vi "Multi_Emitter_transmitter_ui.vi"() -> ()   [LabVIEW 2021]
uses:
  <vilib>/userdefined/High Color/nirio_resource_hc.ctl
  random_limits.ctl
  emitter params.ctl
  mode_type.ctl
  secnario config.ctl
  <instrlib>/niUsrpRio/Config/v1/Host/Public/niUsrpRio Session.ctl
  <instrlib>/_niInstr/Register Bus/v0/Host/Public/Register Bus Session.ctl
  <instrlib>/_niInstr/Register Bus/v0/Host/Private/Session Data.ctl
  <instrlib>/niUsrpRio/Config/v1/Host/Private/DB Queue Reference.ctl
  <instrlib>/niUsrpRio/Config/v1/Host/Private/Daughterboard Data.ctl
  <instrlib>/niUsrpRio/Config/v1/Host/Private/ATR state data.ctl
  <instrlib>/niUsrpRio/Config/v1/Host/Private/Antenna Configuration.ctl
  <instrlib>/niUsrpRio/Config/v1/Host/Private/CPLD Power Mode.ctl
  <instrlib>/niUsrpRio/Config/v1/Host/Public/EEPROM Header.ctl
  <instrlib>/niUsrpRio/Config/v1/Host/Public/EEPROM Device Data Header.ctl
  <instrlib>/niUsrpRio/Config/v1/Host/Public/EEPROM Characterization Header.ctl
  <instrlib>/niUsrpRio/Config/v1/Host/Public/Characterization Data.ctl
  <instrlib>/niUsrpRio/Config/v1/Host/Public/IQ Imbalance.ctl
  <instrlib>/niUsrpRio/Config/v1/Host/niUsrpRio Config v1 Host.lvlib
  <instrlib>/_niInstr/Register Bus/v0/Host/niInstr Register Bus v0 Host.lvlib
panel:
  out "String":string="Transmitting"
  in  "stop":bool=TRUE
  out "Pulse transmited":u32=20 format="%#.1p"
  out "FPGA clock":dbl=0.00084621 format="%#.1g"
  out "lost sampels - P2P":u32
  in  "Tab Control 2":enum32{"RF", "FPGA device", "VST", "TDMS files"}(tab)=enum."TDMS files"
  in  "RF gain":dbl=10.0 min=-130.0 max=30.0 format="%#.8p"
  in  "Center frequency (Hz)":dbl=1600000000.0 format="%#.8p"
  in  "P2P sample rate":dbl=200000000.0 format="%#.8p"
  in  "gen for DF":bool=TRUE
  in  "devicess":T1[](array[typedef])=["IF_transiver_0", "IF_transiver_1", "IF_transiver_2"]
  in  "vst_device":refnum<k15>[](array[refnum])
  in  "file paths":path[](array[path])=[path "C:/Users/PXIe8108_Demo/Documents/CHAIM DATA/chaim/5785_sync_for_elbit/data/pdw_test_file.tdms", path "C:/Users/PXIe8108_Demo/Documents/CHAIM DATA/chaim/5785_sync_for_elbit/data/pdw_test_file_1.tdms", path "C:/Users/PXIe8108_Demo/Documents/CHAIM DATA/chaim/5785_sync_for_elbit/data/pdw_test_file_2.tdms", path "C:/Users/PXIe8108_Demo/Documents/CHAIM DATA/chaim/5785_sync_for_elbit/data/pdw_test_file_3.tdms", path "C:/Users/PXIe8108_Demo/Documents/CHAIM DATA/chaim/5785_sync_for_elbit/data/pdw_test_file_4.tdms"]
  in  "Tab Control":T2(tab)=enum."Present scenario"
  in  "Tab Control 3":T3(tab)
  in  "rand limits":T4={"# Number of emitters"=84, "# Number of frequency per emitter"={"Numeric"=0, "Numeric"=22}, "Frequency range"={"Numeric"=158778625.95419848, "Numeric"=2894656488.5496182}, "Frequency dispersion for each emitter"={"Numeric"=0.0, "Numeric"=1181732.2396298076}, "PRI range (Hz)"={"Numeric"=33.59056776941936, "Numeric"=576.0533087800792}, "Duty cycle - pulse in PRI"={"Numeric"=0.026717557251908396, "Numeric"=0.11832061068702289}, "Amplitude (dB)"={"Numeric"=-34.62595419847328, "Numeric"=-51.11450381679389}, "Modulation depth"={"Numeric"=19162.08437325717, "Numeric"=1181732.2396298076}, "CW"=TRUE, "LFM"=TRUE, "DOA (DEG)"={"Numeric"=0.0, "Numeric"=1181732.2396298076}, "start time (Sec)"=0.0, "end time (Sec)"=50.0, "BPSK"=TRUE, "QPSK"=TRUE} {"DOA (DEG)" scale=0.0..360.0 scale format="%#_6f"; "Modulation depth" scale=1000.0..10000000.0 scale format="%#_6pHz"; "Amplitude (dB)" scale format="%#_6fdB"; "Duty cycle - pulse in PRI" scale=0.0..1.0 scale format="%#_6f"; "PRI range (Hz)" scale=1.0..3000.0 scale format="%#_6pHz"; "Frequency dispersion for each emitter" scale=1000000.0..100000000.0 scale format="%#_6pHz"; "Frequency range" scale=0.0..3200000000.0 scale format="%#_4pHz"; "# Number of frequency per emitter" scale=0.01..3000.0; "# Number of emitters" scale=0.0..200.0}
  in  "array":T5[](array[typedef]) {"t end" format="%#_13g"; "t start" format="%#_13g"; "DOA" format="%#_13g"; "mod depth" format="%#_13pHz"; "amp (dB)" format="%#_13gdB"; "d.c." format="%#_13g"; "hop rate (Hz)" format="%#_13pHz"; "f set" format="%#_6pHz"}
  in  "CSV pulse istraction file in":path=path "C:/Users/PXIe8108_Demo/Documents/CHAIM DATA/chaim/5785_sync_for_elbit/data/pdw_test_file_1.tdms"
  in  "Max number of pulses to present":dbl=500.0
  out "XY Graph":cluster{dbl[], dbl[]}[](graph)=[{[1580800140.0831814, 1580834407.004329], [6.623e-05, 0.00030966]}, {[2383313491.167746, 2383313491.167746], [9.1475e-05, 0.00041018]}, {[196157871.7414, 196805210.53311396], [0.000129485, 0.00029614500000000005]}, {[2893890730.2313623, 2893890730.2313623], [0.00020334, 0.000442945]}, {[2274621870.692988, 2274833527.2774396], [0.000263365, 0.00034213500000000003]}, {[826892720.0215597, 826892720.0215597, 826856448.7121654, 826856448.7121654, 826892720.0215597], [0.00034249, 0.000492215, 0.000492215, 0.00034249, 0.00034249]}, {[1739036854.6760328, 1739036854.6760328], [0.00034619, 0.000488535]}, {[1631334018.3591099, 1631334018.3591099, 1630358408.6030123, 1630358408.6030123, 1631334018.3591099], [0.000347855, 0.000533475, 0.000533475, 0.000347855, 0.000347855]}, {[2708416399.3761177, 2708416399.3761177, 2707616399.3761177, 2707616399.3761177, 2708416399.3761177], [0.00037931, 0.00062138, 0.00062138, 0.00037931, 0.00037931]}, {[2721351197.2689962, 2721351197.2689962, 2720538189.138915, 2720538189.138915, 2721351197.2689962], [0.000498795, 0.00067544, 0.00067544, 0.000498795, 0.000498795]}, {[680656193.5764762, 680656193.5764762], [0.000538285, 0.00082268]}, {[1109531948.6082644, 1109847037.660461], [0.000556095, 0.000896965]}, {[649464539.7076397, 649464539.7076397], [0.000556285, 0.000904715]}, {[2296419656.6224246, 2296419656.6224246], [0.000587275, 0.000693175]}, {[285702284.61423993, 285848939.51949644], [0.00059919, 0.00067695]}, {[1664070770.7339468, 1664070770.7339468, 1663177913.5910895, 1663177913.5910895, 1664070770.7339468], [0.000603985, 0.000816455, 0.000816455, 0.000603985, 0.000603985]}, {[1468598375.6912947, 1468823255.9824655], [0.000646, 0.000855]}, {[2866140899.355443, 2866140899.355443, 2866111509.201144, 2866111509.201144, 2866140899.355443], [0.00074212, 0.001017615, 0.001017615, 0.00074212, 0.00074212]}, {[1368139375.4725895, 1368139375.4725895, 1367154153.7977128, 1367154153.7977128, 1368139375.4725895], [0.000760645, 0.0009064850000000001, 0.0009064850000000001, 0.000760645, 0.000760645]}, {[2603761234.0340424, 2603761234.0340424, 2603302518.4377117, 2603302518.4377117, 2603761234.0340424], [0.00084391, 0.0009991, 0.0009991, 0.00084391, 0.00084391]}, {[472591034.81729984, 472591034.81729984, 472243208.73034334, 472243208.73034334, 472591034.81729984], [0.00086232, 0.00102511, 0.00102511, 0.00086232, 0.00086232]}, {[2879515070.2265687, 2879515070.2265687], [0.000892085, 0.0009666900000000001]}, {[1930031751.255956, 1930634378.2083786], [0.000947115, 0.001243875]}, {[2544253790.7099447, 2544253790.7099447], [0.000951505, 0.0010972]}, {[1824977446.8380158, 1824977446.8380158, 1823987347.828115, 1823987347.828115, 1824977446.8380158], [0.000955035, 0.00103088, 0.00103088, 0.000955035, 0.000955035]}, {[2202964376.3055444, 2202964376.3055444, 2202186166.1888127, 2202186166.1888127, 2202964376.3055444], [0.0009579, 0.001077815, 0.001077815, 0.0009579, 0.0009579]}, {[1514007725.1357243, 1514007725.1357243, 1513539341.060783, 1513539341.060783, 1514007725.1357243], [0.00098325, 0.001212565, 0.001212565, 0.00098325, 0.00098325]}, {[1450681049.292892, 1450681049.292892, 1450119251.5400832, 1450119251.5400832, 1450681049.292892], [0.00101241, 0.0012355, 0.0012355, 0.00101241, 0.00101241]}, {[2681398475.993289, 2681398475.993289, 2680255618.8504314, 2680255618.8504314, 2681398475.993289], [0.001092585, 0.00117186, 0.00117186, 0.001092585, 0.001092585]}, {[1407325102.8832715, 1407650065.0646722], [0.00117266, 0.001376915]}, {[646502856.5768648, 646502856.5768648], [0.00125212, 0.00135483]}, {[1489552387.630272, 1489552387.630272], [0.001275415, 0.001473835]}, {[1592242637.762581, 1592242637.762581], [0.00130457, 0.001472255]}, {[2395186268.257005, 2395186268.257005, 2394895570.582587, 2394895570.582587, 2395186268.257005], [0.00131468, 0.00202553, 0.00202553, 0.00131468, 0.00131468]}, {[894570399.7736647, 894570399.7736647, 893506569.9864306, 893506569.9864306, 894570399.7736647], [0.001317945, 0.001874215, 0.001874215, 0.001317945, 0.001317945]}, {[1705881079.1196365, 1705881079.1196365, 1705857272.4299567, 1705857272.4299567, 1705881079.1196365], [0.001409715, 0.00157576, 0.00157576, 0.001409715, 0.001409715]}, {[2251811039.783873, 2251811039.783873, 2251465616.6405225, 2251465616.6405225, 2251811039.783873], [0.001418575, 0.0014936700000000001, 0.0014936700000000001, 0.001418575, 0.001418575]}, {[2401581298.9745655, 2401646895.871443], [0.00142865, 0.001685845]}, {[549553368.0452126, 549553368.0452126], [0.00145178, 0.00166124]}, {[2845740333.033058, 2845740333.033058, 2845069192.093461, 2845069192.093461, 2845740333.033058], [0.0014714, 0.001763465, 0.001763465, 0.0014714, 0.0014714]}, {[997439632.3541692, 997439632.3541692, 997284833.5925595, 997284833.5925595, 997439632.3541692], [0.0015398, 0.001599625, 0.001599625, 0.0015398, 0.0015398]}, {[740736791.4399742, 740959489.4445376], [0.00172415, 0.00189051]}, {[1442023755.261369, 1442023755.261369, 1440954236.5447915, 1440954236.5447915, 1442023755.261369], [0.0017555, 0.0018244749999999999, 0.0018244749999999999, 0.0017555, 0.0017555]}, {[1449379123.164526, 1449379123.164526, 1449227031.9097729, 1449227031.9097729, 1449379123.164526], [0.00178903, 0.0019603900000000002, 0.0019603900000000002, 0.00178903, 0.00178903]}, {[2151473509.0573254, 2152401104.397768], [0.0017976, 0.0019175249999999998]}, {[771759513.8533624, 772735054.2043267], [0.00181764, 0.00195174]}, {[734571862.4124402, 734571862.4124402], [0.001888725, 0.00207308]}, {[196434462.20135283, 197081800.9930668], [0.001936905, 0.002103565]}, {[2800033039.6975074, 2800033039.6975074], [0.001991115, 0.002089685]}, {[1037674689.0691891, 1037674689.0691891, 1037232211.1930828, 1037232211.1930828, 1037674689.0691891], [0.0022019, 0.0023216350000000003, 0.0023216350000000003, 0.0022019, 0.0022019]}, {[1739062096.239286, 1739062096.239286], [0.002213105, 0.00235545]}, {[348761421.06253767, 348761421.06253767, 347856443.68697214, 347856443.68697214, 348761421.06253767], [0.00221368, 0.00258762, 0.00258762, 0.00221368, 0.00221368]}, {[1925417085.794845, 1925417085.794845], [0.00224428, 0.0025514]}, {[2774160892.4472075, 2774160892.4472075], [0.00226447, 0.0024049600000000003]}, {[2274272054.817277, 2274483711.4017286], [0.00226901, 0.0023477800000000003]}, {[592303104.7088935, 592303104.7088935, 591153679.4215372, 591153679.4215372, 592303104.7088935], [0.002297105, 0.002712025, 0.002712025, 0.002297105, 0.002297105]}, {[2296457382.3406115, 2296457382.3406115], [0.00232635, 0.00243225]}, {[1631268767.3701253, 1631268767.3701253, 1630293157.6140277, 1630293157.6140277, 1631268767.3701253], [0.00237092, 0.00255654, 0.00255654, 0.00237092, 0.00237092]}, {[1737912209.7280185, 1737912209.7280185, 1737388649.5185945, 1737388649.5185945, 1737912209.7280185], [0.00240274, 0.00291464, 0.00291464, 0.00240274, 0.00240274]}, {[1580608219.0446887, 1580642485.9658363], [0.002404205, 0.0026476349999999997]}, {[2721331571.011342, 2721331571.011342, 2720518562.881261, 2720518562.881261, 2721331571.011342], [0.0024361, 0.002612745, 0.002612745, 0.0024361, 0.0024361]}, {[1684929790.2362854, 1684929790.2362854, 1684531383.8617835, 1684531383.8617835, 1684929790.2362854], [0.002441555, 0.0026711900000000004, 0.0026711900000000004, 0.002441555, 0.002441555]}, {[1409155349.303642, 1409155349.303642, 1408497454.5667999, 1408497454.5667999, 1409155349.303642], [0.00252089, 0.002924655, 0.002924655, 0.00252089, 0.00252089]}, {[472660746.49775314, 472660746.49775314, 472312920.41079664, 472312920.41079664, 472660746.49775314], [0.00261325, 0.00277604, 0.00277604, 0.00261325, 0.00261325]}, {[2544181526.819716, 2544181526.819716], [0.00270404, 0.002849735]}, {[2893798188.6703253, 2893798188.6703253], [0.00271437, 0.0029539749999999997]}, {[1063127836.7713614, 1063127836.7713614, 1063048785.3879621, 1063048785.3879621, 1063127836.7713614], [0.002715655, 0.00316565, 0.00316565, 0.002715655, 0.002715655]}, {[2879351416.449822, 2879351416.449822], [0.002725625, 0.0028002300000000003]}, {[191171643.50208235, 191171643.50208235, 190384241.927279, 190384241.927279, 191171643.50208235], [0.00278627, 0.003685405, 0.003685405, 0.00278627, 0.00278627]}, {[1367987460.759361, 1367987460.759361, 1367002239.084484, 1367002239.084484, 1367987460.759361], [0.00280891, 0.00295475, 0.00295475, 0.00280891, 0.00280891]}, {[1824780231.2217734, 1824780231.2217734, 1823790132.2118726, 1823790132.2118726, 1824780231.2217734], [0.002821275, 0.00289712, 0.00289712, 0.002821275, 0.002821275]}, {[2880535219.9598703, 2880535219.9598703], [0.003022575, 0.003540315]}, {[285702284.61423993, 285848939.51949644], [0.00302315, 0.00310091]}, {[1513974483.6750598, 1513974483.6750598, 1513506099.6001184, 1513506099.6001184, 1513974483.6750598], [0.003061055, 0.00329037, 0.00329037, 0.003061055, 0.003061055]}, {[1468527568.6407409, 1468752448.9319117], [0.003138895, 0.003347895]}, {[1705219936.9474678, 1705219936.9474678, 1705196130.257788, 1705196130.257788, 1705219936.9474678], [0.003268275, 0.0034343200000000003, 0.0034343200000000003, 0.003268275, 0.003268275]}, {[1450726250.7121127, 1450726250.7121127, 1450164452.9593036, 1450164452.9593036, 1450726250.7121127], [0.003349665, 0.003572755, 0.003572755, 0.003349665, 0.003349665]}, {[1592373712.2870533, 1592373712.2870533], [0.003379285, 0.00354697]}, {[2202953811.6672707, 2202953811.6672707, 2202175601.550539, 2202175601.550539, 2202953811.6672707], [0.003414445, 0.00353436, 0.00353436, 0.003414445, 0.003414445]}, {[767132097.2802391, 767132097.2802391], [0.00341494, 0.00354653]}, {[1407300380.5714734, 1407625342.7528741], [0.003418365, 0.00362262]}, {[1663727218.3677917, 1663727218.3677917, 1662834361.2249343, 1662834361.2249343, 1663727218.3677917], [0.003432045, 0.003644515, 0.003644515, 0.003432045, 0.003432045]}, {[646535048.6960233, 646535048.6960233], [0.00347894, 0.0035816499999999996]}, {[2501631196.736514, 2501631196.736514, 2500683329.437936, 2500683329.437936, 2501631196.736514], [0.00352081, 0.004239565, 0.004239565, 0.00352081, 0.00352081]}, {[2603498435.1787024, 2603498435.1787024, 2603039719.5823717, 2603039719.5823717, 2603498435.1787024], [0.003578685, 0.0037338749999999998, 0.0037338749999999998, 0.003578685, 0.003578685]}, {[576427464.193527, 576427464.193527, 576181461.7335024, 576181461.7335024, 576427464.193527], [0.00358565, 0.004468335, 0.004468335, 0.00358565, 0.00358565]}, {[771327416.7103804, 772302957.0613447], [0.003643325, 0.003777425]}, {[2681146361.145378, 2681146361.145378, 2680003504.0025215, 2680003504.0025215, 2681146361.145378], [0.00369744, 0.0037767150000000004, 0.0037767150000000004, 0.00369744, 0.00369744]}, {[997064784.9392573, 997064784.9392573, 996909986.1776475, 996909986.1776475, 997064784.9392573], [0.00370627, 0.0037660949999999997, 0.0037660949999999997, 0.00370627, 0.00370627]}, {[1441877832.6486635, 1441877832.6486635, 1440808313.932086, 1440808313.932086, 1441877832.6486635], [0.003709485, 0.0037784600000000004, 0.0037784600000000004, 0.003709485, 0.003709485]}, {[1184679216.2804806, 1184679216.2804806, 1184560662.6349561, 1184560662.6349561, 1184679216.2804806], [0.003714075, 0.003895875, 0.003895875, 0.003714075, 0.003714075]}, {[549553368.0452126, 549553368.0452126], [0.00371751, 0.00392697]}, {[2865958264.9593143, 2865958264.9593143, 2865928874.8050165, 2865928874.8050165, 2865958264.9593143], [0.00372947, 0.004004965, 0.004004965, 0.00372947, 0.00372947]}, {[196469763.70549965, 197117102.4972136], [0.00374432, 0.0039109800000000005]}, {[1449313379.2357452, 1449313379.2357452, 1449161287.9809923, 1449161287.9809923, 1449313379.2357452], [0.003774055, 0.003945415, 0.003945415, 0.003774055, 0.003774055]}, {[2252044360.969656, 2252044360.969656, 2251698937.8263054, 2251698937.8263054, 2252044360.969656], [0.003835815, 0.00391091, 0.00391091, 0.003835815, 0.003835815]}, {[2754483678.838529, 2754483678.838529, 2753805712.736834, 2753805712.736834, 2754483678.838529], [0.00384677, 0.004098795, 0.004098795, 0.00384677, 0.00384677]}, {[952948653.5105207, 952948653.5105207], [0.003865105, 0.004472745]}, {[2151381942.365458, 2152309537.7059007], [0.0039314, 0.004051325]}, {[2383187284.4591317, 2383187284.4591317], [0.00394438, 0.004263085]}, {[2296696866.079333, 2296696866.079333], [0.00406542, 0.00417132]}, {[1739061006.477425, 1739061006.477425], [0.00408002, 0.0042223650000000005]}, {[826977891.3539693, 826977891.3539693, 826941620.044575, 826941620.044575, 826977891.3539693], [0.004121665, 0.00427139, 0.00427139, 0.004121665, 0.004121665]}, {[734773527.9249377, 734773527.9249377], [0.00414752, 0.004331875]}, {[740723871.5179688, 740946569.5225322], [0.004163125, 0.004329485]}, {[2708532448.1508884, 2708532448.1508884, 2707732448.1508884, 2707732448.1508884, 2708532448.1508884], [0.00421376, 0.00445583, 0.00445583, 0.00421376, 0.00421376]}, {[2800458079.9117093, 2800458079.9117093], [0.00423334, 0.0043319100000000004]}, {[2274666375.3677125, 2274878031.952164], [0.00427466, 0.004353429999999999]}, {[1930166193.4840126, 1930768820.4364355], [0.00435341, 0.00465017]}, {[472726219.80381584, 472726219.80381584, 472378393.71685934, 472378393.71685934, 472726219.80381584], [0.004364175, 0.004526965, 0.004526965, 0.004364175, 0.004364175]}, {[513973938.6140039, 513973938.6140039, 513160930.4839227, 513160930.4839227, 513973938.6140039], [0.00437234, 0.00503197, 0.00503197, 0.00437234, 0.00437234]}, {[2720887898.354795, 2720887898.354795, 2720074890.224714, 2720074890.224714, 2720887898.354795], [0.004373405, 0.00455005, 0.00455005, 0.004373405, 0.004373405]}, {[1631196040.4311666, 1631196040.4311666, 1630220430.675069, 1630220430.675069, 1631196040.4311666], [0.004393985, 0.0045796050000000005, 0.0045796050000000005, 0.004393985, 0.004393985]}, {[2544196925.447932, 2544196925.447932], [0.004456575, 0.00460227]}, {[2879644419.775343, 2879644419.775343], [0.004559165, 0.00463377]}, {[648876109.0898465, 648876109.0898465, 648365905.0082139, 648365905.0082139, 648876109.0898465], [0.00460361, 0.0053656400000000005, 0.0053656400000000005, 0.00460361, 0.00460361]}, {[1109802779.3598022, 1110117868.4119987], [0.0046591, 0.00499997]}, {[1824895450.5609894, 1824895450.5609894, 1823905351.5510883, 1823905351.5510883, 1824895450.5609894], [0.00468751, 0.0047633549999999995, 0.0047633549999999995, 0.00468751, 0.00468751]}, {[1580945890.5906582, 1580980157.5118058], [0.004742185, 0.0049856150000000005]}, {[1437976628.2282147, 1437976628.2282147, 1437095570.9594924, 1437095570.9594924, 1437976628.2282147], [0.00476518, 0.005106085, 0.005106085, 0.00476518, 0.00476518]}, {[1367912019.2469618, 1367912019.2469618, 1366926797.572085, 1366926797.572085, 1367912019.2469618], [0.00485718, 0.00500302, 0.00500302, 0.00485718, 0.00485718]}, {[2642546476.6451225, 2642546476.6451225], [0.005085275, 0.005440550000000001]}, {[2401764599.7099066, 2401830196.606784], [0.00512136, 0.005378555]}, {[1706050956.0580258, 1706050956.0580258, 1706027149.368346, 1706027149.368346, 1706050956.0580258], [0.00512683, 0.005292875, 0.005292875, 0.00512683, 0.00512683]}, {[1684720808.2794032, 1684720808.2794032, 1684322401.9049013, 1684322401.9049013, 1684720808.2794032], [0.00513206, 0.005361695, 0.005361695, 0.00513206, 0.00513206]}, {[1513882285.9166286, 1513882285.9166286, 1513413901.8416872, 1513413901.8416872, 1513882285.9166286], [0.00513886, 0.005368175, 0.005368175, 0.00513886, 0.00513886]}, {[2549489795.642293, 2549489795.642293, 2549255329.0537815, 2549255329.0537815, 2549489795.642293], [0.00521551, 0.005773825, 0.005773825, 0.00521551, 0.00521551]}, {[2893775785.8287454, 2893775785.8287454], [0.005225405, 0.00546501]}, {[1925417085.794845, 1925417085.794845], [0.00527129, 0.00557841]}, {[2773799782.619938, 2773799782.619938], [0.005372855, 0.005513345]}, {[285702284.61423993, 285848939.51949644], [0.005447115, 0.005524874999999999]}, {[1591792582.9263594, 1591792582.9263594], [0.005454, 0.0056216849999999995]}, {[771543002.2032365, 772518542.5542008], [0.005469015, 0.005603115]}, {[1662007237.9519308, 1662007237.9519308, 1661585297.023661, 1661585297.023661, 1662007237.9519308], [0.005534915, 0.005872784999999999, 0.005872784999999999, 0.005534915, 0.005534915]}, {[196056287.52977967, 196703626.32149363], [0.005551735, 0.005718395]}, {[1037437198.7534403, 1037437198.7534403, 1036994720.877334, 1036994720.877334, 1037437198.7534403], [0.005624565, 0.0057443, 0.0057443, 0.005624565, 0.005624565]}, {[1469056690.8281426, 1469281571.1193135], [0.00563179, 0.00584079]}, {[1441880281.2689369, 1441880281.2689369, 1440810762.5523593, 1440810762.5523593, 1441880281.2689369], [0.00566347, 0.005732445, 0.005732445, 0.00566347, 0.00566347]}, {[1407344576.5288398, 1407669538.7102404], [0.00566407, 0.005868325000000001]}, {[1450710289.7500644, 1450710289.7500644, 1450148491.9972553, 1450148491.9972553, 1450710289.7500644], [0.00568692, 0.00591001, 0.00591001, 0.00568692, 0.00568692]}, {[646220455.0854722, 646220455.0854722], [0.00570576, 0.00580847]}, {[1449379123.164526, 1449379123.164526, 1449227031.9097729, 1449227031.9097729, 1449379123.164526], [0.005759075, 0.0059304349999999995, 0.0059304349999999995, 0.005759075, 0.005759075]}, {[2296096376.8515058, 2296096376.8515058], [0.005804495, 0.005910395]}, {[2203062554.686778, 2203062554.686778, 2202284344.5700464, 2202284344.5700464, 2203062554.686778], [0.00587099, 0.005990905, 0.005990905, 0.00587099, 0.00587099]}, {[997192164.9389083, 997192164.9389083, 997037366.1772985, 997037366.1772985, 997192164.9389083], [0.005872745, 0.005932570000000001, 0.005932570000000001, 0.005872745, 0.005872745]}, {[1489463100.0648816, 1489463100.0648816], [0.00588631, 0.00608473]}, {[1738991102.0076396, 1738991102.0076396], [0.005946935, 0.006089280000000001]}, {[1409155349.303642, 1409155349.303642, 1408497454.5667999, 1408497454.5667999, 1409155349.303642], [0.005972975, 0.0063767400000000005, 0.0063767400000000005, 0.005972975, 0.005972975]}, {[549553368.0452126, 549553368.0452126], [0.00598324, 0.0061927]}, {[2151368361.287098, 2152295956.6275406], [0.006065195, 0.00618512]}, {[472451052.26250076, 472451052.26250076, 472103226.17554426, 472103226.17554426, 472451052.26250076], [0.006115105, 0.006277895, 0.006277895, 0.006115105, 0.006115105]}, {[894611310.8512297, 894611310.8512297, 893547481.0639956, 893547481.0639956, 894611310.8512297], [0.00611715, 0.00667342, 0.00667342, 0.00611715, 0.00611715]}, {[2544312914.5976286, 2544312914.5976286], [0.00620911, 0.006354805000000001]}, {[2251793159.6009665, 2251793159.6009665, 2251447736.457616, 2251447736.457616, 2251793159.6009665], [0.00625305, 0.006328144999999999, 0.006328144999999999, 0.00625305, 0.00625305]}, {[1663706181.7369223, 1663706181.7369223, 1662813324.5940652, 1662813324.5940652, 1663706181.7369223], [0.00626011, 0.00647258, 0.00647258, 0.00626011, 0.00626011]}, {[2274457073.9342976, 2274668730.518749], [0.006280305, 0.006359075]}, {[2681119550.8547864, 2681119550.8547864, 2679976693.7119293, 2679976693.7119293, 2681119550.8547864], [0.006302295, 0.0063815700000000005, 0.0063815700000000005, 0.006302295, 0.006302295]}, {[2721608626.7745028, 2721608626.7745028, 2720795618.6444216, 2720795618.6444216, 2721608626.7745028], [0.006310705, 0.006487349999999999, 0.006487349999999999, 0.006310705, 0.006310705]}, {[2603629941.7925797, 2603629941.7925797, 2603171226.196249, 2603171226.196249, 2603629941.7925797], [0.006313465, 0.006468655, 0.006468655, 0.006313465, 0.006313465]}, {[2232122993.202605, 2232122993.202605, 2231064792.144404, 2231064792.144404, 2232122993.202605], [0.006389155, 0.007933144999999999, 0.007933144999999999, 0.006389155, 0.006389155]}, {[2879383848.0123553, 2879383848.0123553], [0.0063927, 0.0064673050000000004]}, {[680656193.5764762, 680656193.5764762], [0.00639547, 0.006679865]}, {[734464036.7508987, 734464036.7508987], [0.00640632, 0.006590675]}, {[1631325077.6087675, 1631325077.6087675, 1630349467.85267, 1630349467.85267, 1631325077.6087675], [0.00641705, 0.00660267, 0.00660267, 0.00641705, 0.00641705]}, {[2800080381.365308, 2800080381.365308], [0.00647557, 0.00657414]}, {[1824943974.0034225, 1824943974.0034225, 1823953874.9935215, 1823953874.9935215, 1824943974.0034225], [0.006553745, 0.0066295899999999994, 0.0066295899999999994, 0.006553745, 0.006553745]}, {[740729002.861417, 740951700.8659805], [0.006602095, 0.006768455]}, {[592101558.0578947, 592101558.0578947, 590952132.7705383, 590952132.7705383, 592101558.0578947], [0.00665653, 0.00707145, 0.00707145, 0.00665653, 0.00665653]}, {[2866116016.872055, 2866116016.872055, 2866086626.717757, 2866086626.717757, 2866116016.872055], [0.00671682, 0.006992315, 0.006992315, 0.00671682, 0.00671682]}, {[358280471.4209943, 358280471.4209943, 357692236.12687683, 357692236.12687683, 358280471.4209943], [0.00684166, 0.00769989, 0.00769989, 0.00684166, 0.00684166]}, {[1368746211.5180047, 1368746211.5180047, 1367760989.8431277, 1367760989.8431277, 1368746211.5180047], [0.006905445, 0.007051285, 0.007051285, 0.006905445, 0.006905445]}, {[767335940.9524096, 767335940.9524096], [0.006929165, 0.007060755]}, {[1705193072.3917153, 1705193072.3917153, 1705169265.7020354, 1705169265.7020354, 1705193072.3917153], [0.006985385, 0.00715143, 0.00715143, 0.006985385, 0.006985385]}, {[1580759500.4395807, 1580793767.3607285], [0.00708016, 0.0073235900000000005]}, {[1513727389.6331923, 1513727389.6331923, 1513259005.558251, 1513259005.558251, 1513727389.6331923], [0.007216665, 0.00744598, 0.00744598, 0.007216665, 0.007216665]}, {[771474197.2723118, 772449737.6232761], [0.0072947, 0.0074288]}, {[196593060.32748413, 197240399.11919808], [0.007359155, 0.007525815]}, {[1063299761.3303311, 1063299761.3303311, 1063220709.9469318, 1063220709.9469318, 1063299761.3303311], [0.00739398, 0.007843975, 0.007843975, 0.00739398, 0.00739398]}, {[2395319994.632628, 2395319994.632628, 2395029296.958209, 2395029296.958209, 2395319994.632628], [0.007472035, 0.008182885, 0.008182885, 0.007472035, 0.007472035]}, {[1591840538.1910703, 1591840538.1910703], [0.007528715, 0.0076964]}, {[2296089760.628729, 2296089760.628729], [0.00754357, 0.00764947]}, {[2845678014.9449577, 2845678014.9449577, 2845006874.0053606, 2845006874.0053606, 2845678014.9449577], [0.0075644, 0.007856465, 0.007856465, 0.0075644, 0.0075644]}, {[1442860787.5168386, 1442860787.5168386, 1441791268.800261, 1441791268.800261, 1442860787.5168386], [0.007617455, 0.00768643, 0.00768643, 0.007617455, 0.007617455]}, {[2893859155.9198585, 2893859155.9198585], [0.007736435, 0.00797604]}, {[1449313379.2357452, 1449313379.2357452, 1449161287.9809923, 1449161287.9809923, 1449313379.2357452], [0.007744095, 0.007915455, 0.007915455, 0.007744095, 0.007744095]}, {[1929892018.70746, 1930494645.6598828], [0.007759705, 0.008056465]}, {[2383333327.4941196, 2383333327.4941196], [0.007797285, 0.00811599]}, {[1738987303.8463974, 1738987303.8463974], [0.00781385, 0.007956195000000001]}, {[1684959175.0429544, 1684959175.0429544, 1684560768.6684525, 1684560768.6684525, 1684959175.0429544], [0.007822565, 0.0080522, 0.0080522, 0.007822565, 0.007822565]}, {[472589383.96592045, 472589383.96592045, 472241557.87896395, 472241557.87896395, 472589383.96592045], [0.00786603, 0.008028819999999999, 0.008028819999999999, 0.00786603, 0.00786603]}, {[285702284.61423993, 285848939.51949644], [0.007871075, 0.007948835]}, {[826842646.1959547, 826842646.1959547, 826806374.8865603, 826806374.8865603, 826842646.1959547], [0.00790084, 0.008050564999999999, 0.008050564999999999, 0.00790084, 0.00790084]}, {[1407289616.8067927, 1407614578.9881935], [0.00790977, 0.008114025]}, {[646574240.5246942, 646574240.5246942], [0.007932575, 0.008035285000000001]}, {[2544396206.6976385, 2544396206.6976385], [0.00796164, 0.008107335]}, {[1450589789.1001937, 1450589789.1001937, 1450027991.3473847, 1450027991.3473847, 1450589789.1001937], [0.008024175, 0.008247265, 0.008247265, 0.008024175, 0.008024175]}, {[997068963.0170933, 997068963.0170933, 996914164.2554835, 996914164.2554835, 997068963.0170933], [0.00803922, 0.008099045, 0.008099045, 0.00803922, 0.00803922]}, {[1184681571.1905012, 1184681571.1905012, 1184563017.5449767, 1184563017.5449767, 1184681571.1905012], [0.00804374, 0.00822554, 0.00822554, 0.00804374, 0.00804374]}, {[2708441543.4714837, 2708441543.4714837, 2707641543.4714837, 2707641543.4714837, 2708441543.4714837], [0.00804821, 0.00829028, 0.00829028, 0.00804821, 0.00804821]}, {[1468945567.8784726, 1469170448.1696434], [0.00812469, 0.008333690000000001]}, {[2317953472.4606924, 2317953472.4606924], [0.008127065, 0.010070595]}, {[2151428965.0152593, 2152356560.355702], [0.008198995, 0.00831892]}, {[348658294.97384024, 348658294.97384024, 347753317.5982747, 347753317.5982747, 348658294.97384024], [0.00822505, 0.008598989999999999, 0.008598989999999999, 0.00822505, 0.00822505]}, {[2879290525.343538, 2879290525.343538], [0.00822624, 0.008300845]}, {[2721648319.4452286, 2721648319.4452286, 2720835311.3151474, 2720835311.3151474, 2721648319.4452286], [0.00824801, 0.008424655, 0.008424655, 0.00824801, 0.00824801]}, {[549553368.0452126, 549553368.0452126], [0.008248965, 0.008458425]}, {[2274181451.318759, 2274393107.9032106], [0.008285955, 0.008364725]}, {[1925417085.794845, 1925417085.794845], [0.008298295, 0.008605415]}, {[2203696245.445428, 2203696245.445428, 2202918035.3286963, 2202918035.3286963, 2203696245.445428], [0.00832753, 0.008447445, 0.008447445, 0.00832753, 0.00832753]}, {[2234822554.778743, 2234822554.778743, 2233967853.9240417, 2233967853.9240417, 2234822554.778743], [0.00838687, 0.009563084999999999, 0.009563084999999999, 0.00838687, 0.00838687]}, {[1824774748.6669872, 1824774748.6669872, 1823784649.6570861, 1823784649.6570861, 1824774748.6669872], [0.00841998, 0.008495825, 0.008495825, 0.00841998, 0.00841998]}, {[1631352666.923056, 1631352666.923056, 1630377057.1669583, 1630377057.1669583, 1631352666.923056], [0.008440115, 0.008625734999999999, 0.008625734999999999, 0.008440115, 0.008440115]}, {[2774131413.6681013, 2774131413.6681013], [0.00848124, 0.00862173]}, {[2880970854.8082085, 2880970854.8082085], [0.008508115, 0.009025855]}, {[734700021.0995475, 734700021.0995475], [0.008665115, 0.00884947]}, {[2252003552.7850003, 2252003552.7850003, 2251658129.6416497, 2251658129.6416497, 2252003552.7850003], [0.00867029, 0.008745385000000001, 0.008745385000000001, 0.00867029, 0.00867029]}, {[2800025632.1998563, 2800025632.1998563], [0.008717795, 0.008816365]}, {[1109761244.8834865, 1110076333.935683], [0.00876211, 0.00910298]}, {[2402109882.815182, 2402175479.712059], [0.008814065, 0.00907126]}, {[1705327327.5286741, 1705327327.5286741, 1705303520.8389943, 1705303520.8389943, 1705327327.5286741], [0.00884394, 0.009009985, 0.009009985, 0.00884394, 0.00884394]}, {[2681025969.7430334, 2681025969.7430334, 2679883112.6001763, 2679883112.6001763, 2681025969.7430334], [0.00890715, 0.008986425000000001, 0.008986425000000001, 0.00890715, 0.00890715]}, {[1368691160.8756483, 1368691160.8756483, 1367705939.2007713, 1367705939.2007713, 1368691160.8756483], [0.008953715, 0.009099554999999999, 0.009099554999999999, 0.008953715, 0.008953715]}, {[2755073705.6039343, 2755073705.6039343, 2754395739.502239, 2754395739.502239, 2755073705.6039343], [0.009011195, 0.009263219999999999, 0.009263219999999999, 0.009011195, 0.009011195]}, {[740893521.581745, 741116219.5863085], [0.00904107, 0.00920743]}, {[1037849812.9642878, 1037849812.9642878, 1037407335.0881815, 1037407335.0881815, 1037849812.9642878], [0.009047235, 0.00916697, 0.00916697, 0.009047235, 0.009047235]}, {[2603575983.0110044, 2603575983.0110044, 2603117267.414674, 2603117267.414674, 2603575983.0110044], [0.00904824, 0.00920343, 0.00920343, 0.00904824, 0.00904824]}, {[1663658939.9626198, 1663658939.9626198, 1662766082.8197625, 1662766082.8197625, 1663658939.9626198], [0.00908817, 0.009300639999999999, 0.009300639999999999, 0.00908817, 0.00908817]}, {[771369562.2871455, 772345102.6381098], [0.009120385, 0.009254485]}, {[196558768.56656957, 197206107.35828352], [0.00916657, 0.009333230000000001]}, {[2296716536.6770926, 2296716536.6770926], [0.00928264, 0.00938854]}, {[1513642762.6943433, 1513642762.6943433, 1513174378.619402, 1513174378.619402, 1513642762.6943433], [0.009294465, 0.00952378, 0.00952378, 0.009294465, 0.009294465]}, {[1580885021.106201, 1580919288.0273485], [0.009418135, 0.009661564999999999]}, {[1409155349.303642, 1409155349.303642, 1408497454.5667999, 1408497454.5667999, 1409155349.303642], [0.00942506, 0.009828825000000001, 0.009828825000000001, 0.00942506, 0.00942506]}, {[1442388293.9242394, 1442388293.9242394, 1441318775.2076619, 1441318775.2076619, 1442388293.9242394], [0.00957144, 0.009640415000000001, 0.009640415000000001, 0.00957144, 0.00957144]}, {[1592106085.5720952, 1592106085.5720952], [0.00960343, 0.009771115]}, {[472872663.51137424, 472872663.51137424, 472524837.42441773, 472524837.42441773, 472872663.51137424], [0.00961696, 0.00977975, 0.00977975, 0.00961696, 0.00961696]}, {[1739056589.8570004, 1739056589.8570004], [0.009680765, 0.00982311]}, {[2865918129.068333, 2865918129.068333, 2865888738.914035, 2865888738.914035, 2865918129.068333], [0.00970417, 0.009979665, 0.009979665, 0.00970417, 0.00970417]}, {[2544131870.074193, 2544131870.074193], [0.009714175, 0.00985987]}, {[1737963778.3685791, 1737963778.3685791, 1737440218.1591551, 1737440218.1591551, 1737963778.3685791], [0.009719545, 0.010231444999999999, 0.010231444999999999, 0.009719545, 0.009719545]}, {[1449379123.164526, 1449379123.164526, 1449227031.9097729, 1449227031.9097729, 1449379123.164526], [0.009729115, 0.009900475, 0.009900475, 0.009729115, 0.009729115]}, {[953499027.9946896, 953499027.9946896], [0.009734975, 0.010342615]}, {[2879485571.71311, 2879485571.71311], [0.01005978, 0.010134385000000001]}, {[1407325102.8832715, 1407650065.0646722], [0.010155475, 0.010359730000000001]}, {[513660630.55560327, 513660630.55560327, 512847622.4255221, 512847622.4255221, 513660630.55560327], [0.01015609, 0.01081572, 0.01081572, 0.01015609, 0.01015609]}, {[646084411.6524413, 646084411.6524413], [0.010159395, 0.010262105]}, {[2721571531.409893, 2721571531.409893, 2720758523.279812, 2720758523.279812, 2721571531.409893], [0.010185315, 0.01036196, 0.01036196, 0.010185315, 0.010185315]}, {[997428634.6466807, 997428634.6466807, 997273835.8850709, 997273835.8850709, 997428634.6466807], [0.010205695, 0.01026552, 0.01026552, 0.010205695, 0.010205695]}, {[2893835322.437974, 2893835322.437974], [0.010247465, 0.010487070000000001]}, {[1824794220.2309835, 1824794220.2309835, 1823804121.2210824, 1823804121.2210824, 1824794220.2309835], [0.010286215, 0.01036206, 0.01036206, 0.010286215, 0.010286215]}, {[2273952247.704483, 2274163904.2889347], [0.0102916, 0.01037037]}, {[285702284.61423993, 285848939.51949644], [0.01029504, 0.0103728]}, {[2151478147.548687, 2152405742.8891296], [0.010332795, 0.01045272]}, {[1450601418.442362, 1450601418.442362, 1450039620.689553, 1450039620.689553, 1450601418.442362], [0.010361425, 0.010584515000000001, 0.010584515000000001, 0.010361425, 0.010361425]}, {[767010222.9587655, 767010222.9587655], [0.010443385, 0.010574975]}, {[1631375527.8903732, 1631375527.8903732, 1630399918.1342757, 1630399918.1342757, 1631375527.8903732], [0.010463175, 0.010648794999999999, 0.010648794999999999, 0.010463175, 0.010463175]}, {[1489671501.0283628, 1489671501.0283628], [0.01049721, 0.01069563]}, {[1685032737.4106975, 1685032737.4106975, 1684634331.0361953, 1684634331.0361953, 1685032737.4106975], [0.010513065, 0.0107427, 0.0107427, 0.010513065, 0.010513065]}, {[549553368.0452126, 549553368.0452126], [0.010514695, 0.010724154999999999]}, {[1468768186.1909142, 1468993066.482085], [0.010617585, 0.010826585000000001]}, {[649464539.7076397, 649464539.7076397], [0.010647545, 0.010995975]}, {[1705828281.0006616, 1705828281.0006616, 1705804474.3109818, 1705804474.3109818, 1705828281.0006616], [0.010702495, 0.01086854, 0.01086854, 0.010702495, 0.010702495]}, {[2203292231.878026, 2203292231.878026, 2202514021.761295, 2202514021.761295, 2203292231.878026], [0.010784075, 0.01090399, 0.01090399, 0.010784075, 0.010784075]}, {[894381668.9630754, 894381668.9630754, 893317839.1758413, 893317839.1758413, 894381668.9630754], [0.01091636, 0.01147263, 0.01147263, 0.01091636, 0.01091636]}, {[734686923.4632208, 734686923.4632208], [0.01092391, 0.011108265]}, {[771534875.8640743, 772510416.2150387], [0.010946075, 0.011080175]}, {[2800471429.041852, 2800471429.041852], [0.010960025, 0.011058595]}, {[196626663.36879516, 197274002.1605091], [0.010973985, 0.011140645000000001]}, {[1367892214.719479, 1367892214.719479, 1366906993.0446022, 1366906993.0446022, 1367892214.719479], [0.01100198, 0.01114782, 0.01114782, 0.01100198, 0.01100198]}, {[591753124.3896897, 591753124.3896897, 590603699.1023333, 590603699.1023333, 591753124.3896897], [0.011015955, 0.011430874999999998, 0.011430874999999998, 0.011015955, 0.011015955]}, {[2296311292.262669, 2296311292.262669], [0.011021715, 0.011127615]}, {[2252072419.0839663, 2252072419.0839663, 2251726995.9406157, 2251726995.9406157, 2252072419.0839663], [0.011087525, 0.011162620000000002, 0.011162620000000002, 0.011087525, 0.011087525]}, {[1930031751.255956, 1930634378.2083786], [0.011166, 0.01146276]}, {[1925417085.794845, 1925417085.794845], [0.0113253, 0.01163242]}, {[472591034.81729984, 472591034.81729984, 472243208.73034334, 472243208.73034334, 472591034.81729984], [0.011367885, 0.011530674999999999, 0.011530674999999999, 0.011367885, 0.011367885]}, {[1513665052.2554708, 1513665052.2554708, 1513196668.180529, 1513196668.180529, 1513665052.2554708], [0.01137227, 0.011601585000000001, 0.011601585000000001, 0.01137227, 0.01137227]}, {[2544191636.0495725, 2544191636.0495725], [0.01146671, 0.011612405]}, {[740788064.5607747, 741010762.5653381], [0.011480045, 0.011646405]}, {[2681398475.993289, 2681398475.993289, 2680255618.8504314, 2680255618.8504314, 2681398475.993289], [0.011512005, 0.01159128, 0.01159128, 0.011512005, 0.011512005]}, {[1441785058.2562668, 1441785058.2562668, 1440715539.5396893, 1440715539.5396893, 1441785058.2562668], [0.011525425, 0.011594400000000001, 0.011594400000000001, 0.011525425, 0.011525425]}, {[1739041782.8394334, 1739041782.8394334], [0.01154768, 0.011690025]}, {[2773676206.927871, 2773676206.927871], [0.011589625, 0.011730115]}, {[1662122651.5154796, 1662122651.5154796, 1661700710.5872097, 1661700710.5872097, 1662122651.5154796], [0.011627, 0.01196487, 0.01196487, 0.011627, 0.011627]}, {[2383159668.1059523, 2383159668.1059523], [0.01165019, 0.011968895]}, {[1592012680.4076858, 1592012680.4076858], [0.011678145, 0.01184583]}, {[826890425.1105181, 826890425.1105181, 826854153.8011237, 826854153.8011237, 826890425.1105181], [0.01168002, 0.011829745, 0.011829745, 0.01168002, 0.01168002]}, {[1449313379.2357452, 1449313379.2357452, 1449161287.9809923, 1449161287.9809923, 1449313379.2357452], [0.01171414, 0.0118855, 0.0118855, 0.01171414, 0.01171414]}, {[1581070751.4417686, 1581105018.3629162], [0.011756115, 0.011999544999999999]}, {[2603675335.7246003, 2603675335.7246003, 2603216620.12827, 2603216620.12827, 2603675335.7246003], [0.01178302, 0.01193821, 0.01193821, 0.01178302, 0.01178302]}, {[2708163722.6427097, 2708163722.6427097, 2707363722.6427097, 2707363722.6427097, 2708163722.6427097], [0.011882665, 0.012124735000000001, 0.012124735000000001, 0.011882665, 0.011882665]}, {[2879846973.8631067, 2879846973.8631067], [0.01189332, 0.011967925]}, {[1663627126.801152, 1663627126.801152, 1662734269.658295, 1662734269.658295, 1663627126.801152], [0.01191623, 0.0121287, 0.0121287, 0.01191623, 0.01191623]}, {[1063253930.5611609, 1063253930.5611609, 1063174879.1777617, 1063174879.1777617, 1063253930.5611609], [0.012072305, 0.0125223, 0.0125223, 0.012072305, 0.012072305]}, {[2721351197.2689962, 2721351197.2689962, 2720538189.138915, 2720538189.138915, 2721351197.2689962], [0.01212262, 0.012299265, 0.012299265, 0.01212262, 0.01212262]}, {[1824744659.720948, 1824744659.720948, 1823754560.7110472, 1823754560.7110472, 1824744659.720948], [0.01215245, 0.012228295, 0.012228295, 0.01215245, 0.01215245]}, {[680656193.5764762, 680656193.5764762], [0.01225265, 0.012537045]}, {[2274555327.372104, 2274766983.956556], [0.01229725, 0.01237602]}, {[996991553.1942685, 996991553.1942685, 996836754.4326587, 996836754.4326587, 996991553.1942685], [0.012372165, 0.012431989999999999, 0.012431989999999999, 0.012372165, 0.012372165]}, {[1184652956.373427, 1184652956.373427, 1184534402.7279022, 1184534402.7279022, 1184652956.373427], [0.012373405, 0.012555205, 0.012555205, 0.012373405, 0.012373405]}, {[646502856.5768648, 646502856.5768648], [0.012386215, 0.012488925000000001]}, {[1407300380.5714734, 1407625342.7528741], [0.01240118, 0.012605435]}, {[2643010540.7462864, 2643010540.7462864], [0.012452405, 0.01280768]}, {[2151502369.854427, 2152429965.1948695], [0.01246659, 0.012586515]}, {[1037638449.2997943, 1037638449.2997943, 1037195971.423688, 1037195971.423688, 1037638449.2997943], [0.0124699, 0.012589635, 0.012589635, 0.0124699, 0.0124699]}, {[1631390437.082894, 1631390437.082894, 1630414827.3267965, 1630414827.3267965, 1631390437.082894], [0.01248624, 0.012671859999999998, 0.012671859999999998, 0.01248624, 0.01248624]}, {[2401581298.9745655, 2401646895.871443], [0.012506775, 0.01276397]}, {[1705079320.2711687, 1705079320.2711687, 1705055513.581489, 1705055513.581489, 1705079320.2711687], [0.01256105, 0.012727095, 0.012727095, 0.01256105, 0.01256105]}, {[2865887879.658575, 2865887879.658575, 2865858489.5042768, 2865858489.5042768, 2865887879.658575], [0.01269152, 0.012967015, 0.012967015, 0.01269152, 0.01269152]}, {[1450690643.6663926, 1450690643.6663926, 1450128845.9135835, 1450128845.9135835, 1450690643.6663926], [0.01269868, 0.01292177, 0.01292177, 0.01269868, 0.01269868]}, {[285702284.61423993, 285848939.51949644], [0.012719, 0.012796759999999999]}, {[2893895761.2772584, 2893895761.2772584], [0.012758495, 0.0129981]}, {[2296605379.3567424, 2296605379.3567424], [0.012760785, 0.012866685000000001]}, {[771488196.8876398, 772463737.2386041], [0.01277176, 0.01290586]}, {[549553368.0452126, 549553368.0452126], [0.012780425, 0.012989885]}, {[195898497.85518265, 196545836.6468966], [0.012781405, 0.012948065]}, {[1437851190.719583, 1437851190.719583, 1436970133.4508605, 1436970133.4508605, 1437851190.719583], [0.01280003, 0.013140935000000001, 0.013140935000000001, 0.01280003, 0.01280003]}, {[1109829949.8347387, 1110145038.8869352], [0.01286512, 0.01320599]}, {[1409155349.303642, 1409155349.303642, 1408497454.5667999, 1408497454.5667999, 1409155349.303642], [0.01287714, 0.013280905, 0.013280905, 0.01287714, 0.01287714]}, {[1368466421.5023482, 1368466421.5023482, 1367481199.8274713, 1367481199.8274713, 1368466421.5023482], [0.01305025, 0.013196089999999999, 0.013196089999999999, 0.01305025, 0.01305025]}, {[1468372436.7318177, 1468597317.0229886], [0.01311048, 0.013319480000000002]}, {[472660746.49775314, 472660746.49775314, 472312920.41079664, 472312920.41079664, 472660746.49775314], [0.013118815, 0.013281605, 0.013281605, 0.013118815, 0.013118815]}, {[734531669.9672707, 734531669.9672707], [0.013182705, 0.01336706]}, {[2800063313.061628, 2800063313.061628], [0.013202255, 0.013300824999999999]}, {[1684881095.0267966, 1684881095.0267966, 1684482688.6522946, 1684482688.6522946, 1684881095.0267966], [0.01320357, 0.013433205, 0.013433205, 0.01320357, 0.01320357]}, {[2544197911.236506, 2544197911.236506], [0.013219245, 0.013364939999999999]}, {[2203413305.73774, 2203413305.73774, 2202635095.6210084, 2202635095.6210084, 2203413305.73774], [0.013240615, 0.01336053, 0.01336053, 0.013240615, 0.013240615]}, {[1738992369.7666178, 1738992369.7666178], [0.013414595, 0.01355694]}, {[1513716142.7429366, 1513716142.7429366, 1513247758.667995, 1513247758.667995, 1513716142.7429366], [0.013450075, 0.013679390000000001, 0.013679390000000001, 0.013450075, 0.013450075]}, {[1442483137.044008, 1442483137.044008, 1441413618.3274305, 1441413618.3274305, 1442483137.044008], [0.013479405, 0.01354838, 0.01354838, 0.013479405, 0.013479405]}, {[2252200717.2649603, 2252200717.2649603, 2251855294.1216097, 2251855294.1216097, 2252200717.2649603], [0.013504765, 0.013579860000000001, 0.013579860000000001, 0.013504765, 0.013504765]}, {[2395401128.42587, 2395401128.42587, 2395110430.751451, 2395110430.751451, 2395401128.42587], [0.01362939, 0.01434024, 0.01434024, 0.01362939, 0.01362939]}, {[2845598947.8827124, 2845598947.8827124, 2844927806.943115, 2844927806.943115, 2845598947.8827124], [0.0136574, 0.013949465, 0.013949465, 0.0136574, 0.0136574]}, {[1449379123.164526, 1449379123.164526, 1449227031.9097729, 1449227031.9097729, 1449379123.164526], [0.01369916, 0.01387052, 0.01387052, 0.01369916, 0.01369916]}, {[2879515070.2265687, 2879515070.2265687], [0.01372686, 0.013801465]}, {[1592002108.2398193, 1592002108.2398193], [0.01375286, 0.013920545000000001]}, {[740789338.152149, 741012036.1567124], [0.01391902, 0.014085380000000002]}, {[767187636.012659, 767187636.012659], [0.01395761, 0.0140892]}, {[2880502008.4366674, 2880502008.4366674], [0.01399365, 0.014511389999999999]}, {[1824813016.5475392, 1824813016.5475392, 1823822917.5376384, 1823822917.5376384, 1824813016.5475392], [0.01401869, 0.014094535, 0.014094535, 0.01401869, 0.01401869]}, {[2721331571.011342, 2721331571.011342, 2720518562.881261, 2720518562.881261, 2721331571.011342], [0.014059925, 0.014236569999999999, 0.014236569999999999, 0.014059925, 0.014059925]}, {[1581087329.7835996, 1581121596.7047474], [0.01409409, 0.01433752]}, {[2681146361.145378, 2681146361.145378, 2680003504.0025215, 2680003504.0025215, 2681146361.145378], [0.01411686, 0.014196135, 0.014196135, 0.01411686, 0.01411686]}, {[576584119.8246146, 576584119.8246146, 576338117.36459, 576338117.36459, 576584119.8246146], [0.01416452, 0.015047205, 0.015047205, 0.01416452, 0.01416452]}, {[2754772247.5167694, 2754772247.5167694, 2754094281.4150743, 2754094281.4150743, 2754772247.5167694], [0.01417562, 0.014427645, 0.014427645, 0.01417562, 0.01417562]}, {[348761421.06253767, 348761421.06253767, 347856443.68697214, 347856443.68697214, 348761421.06253767], [0.01423642, 0.01461036, 0.01461036, 0.01423642, 0.01423642]}, {[2274583962.178201, 2274795618.762653], [0.0143029, 0.014381670000000001]}, {[1925417085.794845, 1925417085.794845], [0.014352305, 0.014659424999999998]}, {[1705152361.8565383, 1705152361.8565383, 1705128555.1668584, 1705128555.1668584, 1705152361.8565383], [0.014419605, 0.01458565, 0.01458565, 0.014419605, 0.014419605]}, {[2296811450.9059887, 2296811450.9059887], [0.01449986, 0.01460576]}, {[1631161069.0720503, 1631161069.0720503, 1630185459.3159528, 1630185459.3159528, 1631161069.0720503], [0.014509305, 0.014694925, 0.014694925, 0.014509305, 0.014509305]}, {[2603521127.393495, 2603521127.393495, 2603062411.797165, 2603062411.797165, 2603521127.393495], [0.014517795, 0.014672985, 0.014672985, 0.014517795, 0.014517795]}, {[997214126.6378937, 997214126.6378937, 997059327.8762839, 997059327.8762839, 997214126.6378937], [0.01453864, 0.014598465, 0.014598465, 0.01453864, 0.01453864]}, {[1930166193.4840126, 1930768820.4364355], [0.014572295, 0.014869055]}, {[196523707.07466388, 197171045.86637783], [0.01458882, 0.014755480000000001]}, {[771488668.6608338, 772464209.0117981], [0.014597445, 0.014731545]}, {[2151410798.171105, 2152338393.5115476], [0.01460039, 0.014720315]}, {[646535048.6960233, 646535048.6960233], [0.01461303, 0.014715740000000001]}, {[1407344576.5288398, 1407669538.7102404], [0.014646885, 0.01485114]}, {[2773912851.8077908, 2773912851.8077908], [0.01469801, 0.0148385]}, {[1663847804.5114377, 1663847804.5114377, 1662954947.3685806, 1662954947.3685806, 1663847804.5114377], [0.01474429, 0.01495676, 0.01495676, 0.01474429, 0.01474429]}, {[472726219.80381584, 472726219.80381584, 472378393.71685934, 472378393.71685934, 472726219.80381584], [0.01486974, 0.015032529999999999, 0.015032529999999999, 0.01486974, 0.01486974]}, {[2543737771.393944, 2543737771.393944], [0.01497178, 0.015117475]}, {[1450736947.7155507, 1450736947.7155507, 1450175149.9627416, 1450175149.9627416, 1450736947.7155507], [0.015035935, 0.015259025, 0.015259025, 0.015035935, 0.015035935]}, {[549553368.0452126, 549553368.0452126], [0.01504615, 0.01525561]}, {[1368866548.5996418, 1368866548.5996418, 1367881326.9247649, 1367881326.9247649, 1368866548.5996418], [0.015098515, 0.015244355, 0.015244355, 0.015098515, 0.015098515]}, {[1489384229.2247882, 1489384229.2247882], [0.015108105, 0.015306525]}, {[285702284.61423993, 285848939.51949644], [0.015142965, 0.015220725]}, {[190782813.86341596, 190782813.86341596, 189995412.2886126, 189995412.2886126, 190782813.86341596], [0.015215365, 0.0161145, 0.0161145, 0.015215365, 0.015215365]}, {[2893891235.857575, 2893891235.857575], [0.01526953, 0.015509135]}, {[1739070145.3337214, 1739070145.3337214], [0.01528151, 0.015423855]}, {[592569788.5100172, 592569788.5100172, 591420363.2226608, 591420363.2226608, 592569788.5100172], [0.01537538, 0.0157903, 0.0157903, 0.01537538, 0.01537538]}, {[1442768379.7619472, 1442768379.7619472, 1441698861.0453696, 1441698861.0453696, 1442768379.7619472], [0.01543339, 0.015502365, 0.015502365, 0.01543339, 0.01543339]}, {[734571862.4124402, 734571862.4124402], [0.015441505, 0.01562586]}, {[2800033039.6975074, 2800033039.6975074], [0.01544448, 0.01554305]}, {[826971244.5115755, 826971244.5115755, 826934973.2021811, 826934973.2021811, 826971244.5115755], [0.015459195, 0.01560892, 0.01560892, 0.015459195, 0.015459195]}, {[2383588851.664672, 2383588851.664672], [0.015503095, 0.0158218]}, {[1513927073.4151356, 1513927073.4151356, 1513458689.3401942, 1513458689.3401942, 1513927073.4151356], [0.015527875, 0.01575719, 0.01575719, 0.015527875, 0.015527875]}, {[2879351416.449822, 2879351416.449822], [0.0155604, 0.015635005]}, {[1468598375.6912947, 1468823255.9824655], [0.015603375, 0.015812375]}, {[953021686.3875353, 953021686.3875353], [0.015604845, 0.016212485]}, {[2866159419.8354435, 2866159419.8354435, 2866130029.6811447, 2866130029.6811447, 2866159419.8354435], [0.015678865, 0.01595436, 0.01595436, 0.015678865, 0.015678865]}, {[1449313379.2357452, 1449313379.2357452, 1449161287.9809923, 1449161287.9809923, 1449313379.2357452], [0.01568418, 0.015855539999999998, 0.015855539999999998, 0.01568418, 0.01568418]}, {[2203646760.79115, 2203646760.79115, 2202868550.6744184, 2202868550.6744184, 2203646760.79115], [0.01569716, 0.015817075000000003, 0.015817075000000003, 0.01569716, 0.01569716]}, {[894529950.184921, 894529950.184921, 893466120.397687, 893466120.397687, 894529950.184921], [0.01571557, 0.016271840000000003, 0.016271840000000003, 0.01571557, 0.01571557]}, {[2708285940.1411138, 2708285940.1411138, 2707485940.1411138, 2707485940.1411138, 2708285940.1411138], [0.015717115, 0.015959185, 0.015959185, 0.015717115, 0.015717115]}, {[1591707444.1506658, 1591707444.1506658], [0.015827575, 0.01599526]}, {[1824944860.9996355, 1824944860.9996355, 1823954761.9897346, 1823954761.9897346, 1824944860.9996355], [0.015884925, 0.015960770000000003, 0.015960770000000003, 0.015884925, 0.015884925]}, {[1037700241.6664652, 1037700241.6664652, 1037257763.7903589, 1037257763.7903589, 1037700241.6664652], [0.015892565, 0.0160123, 0.0160123, 0.015892565, 0.015892565]}, {[1685010958.8221562, 1685010958.8221562, 1684612552.4476542, 1684612552.4476542, 1685010958.8221562], [0.015894075, 0.01612371, 0.01612371, 0.015894075, 0.015894075]}, {[2502009309.8638086, 2502009309.8638086, 2501061442.5652304, 2501061442.5652304, 2502009309.8638086], [0.015896655, 0.01661541, 0.01661541, 0.015896655, 0.015896655]}, {[2252025990.74781, 2252025990.74781, 2251680567.6044593, 2251680567.6044593, 2252025990.74781], [0.015922, 0.015997095, 0.015997095, 0.015922, 0.015922]}, {[513500939.01757, 513500939.01757, 512687930.88748884, 512687930.88748884, 513500939.01757], [0.015939835, 0.016599465, 0.016599465, 0.015939835, 0.015939835]}, {[2720887898.354795, 2720887898.354795, 2720074890.224714, 2720074890.224714, 2720887898.354795], [0.01599723, 0.016173875, 0.016173875, 0.01599723, 0.01599723]}, {[2401764599.7099066, 2401830196.606784], [0.016199485, 0.01645668]}, {[2296485831.897701, 2296485831.897701], [0.01623893, 0.016344829999999998]}, {[1705177458.648403, 1705177458.648403, 1705153651.958723, 1705153651.958723, 1705177458.648403], [0.01627816, 0.016444205, 0.016444205, 0.01627816, 0.01627816]}, {[2274550427.1853294, 2274762083.769781], [0.016308545, 0.016387315]}, {[1409155349.303642, 1409155349.303642, 1408497454.5667999, 1408497454.5667999, 1409155349.303642], [0.016329225, 0.01673299, 0.01673299, 0.016329225, 0.016329225]}, {[740785332.0616596, 741008030.066223], [0.016357995, 0.016524355]}, {[196467749.96688247, 197115088.75859642], [0.016396235, 0.016562894999999998]}, {[771461928.4980813, 772437468.8490456], [0.016423135, 0.016557235]}, {[1580888728.5910487, 1580922995.5121963], [0.016432065, 0.016675495]}, {[1631219411.9405723, 1631219411.9405723, 1630243802.1844747, 1630243802.1844747, 1631219411.9405723], [0.01653237, 0.016717990000000002, 0.016717990000000002, 0.01653237, 0.01653237]}, {[472451052.26250076, 472451052.26250076, 472103226.17554426, 472103226.17554426, 472451052.26250076], [0.01662067, 0.01678346, 0.01678346, 0.01662067, 0.01662067]}, {[1184475330.874736, 1184475330.874736, 1184356777.2292113, 1184356777.2292113, 1184475330.874736], [0.016703065, 0.016884865, 0.016884865, 0.016703065, 0.016703065]}, {[997330210.8612553, 997330210.8612553, 997175412.0996455, 997175412.0996455, 997330210.8612553], [0.016705115, 0.01676494, 0.01676494, 0.016705115, 0.016705115]}, {[2681119550.8547864, 2681119550.8547864, 2679976693.7119293, 2679976693.7119293, 2681119550.8547864], [0.016721715, 0.016800990000000002, 0.016800990000000002, 0.016721715, 0.016721715]}, {[2543927090.6532555, 2543927090.6532555], [0.01672431, 0.016870005]}, {[2151473509.0573254, 2152401104.397768], [0.01673419, 0.016854115]}, {[1063716334.4449911, 1063716334.4449911, 1063637283.0615919, 1063637283.0615919, 1063716334.4449911], [0.01675063, 0.017200625, 0.017200625, 0.01675063, 0.01675063]}, {[358767166.9186876, 358767166.9186876, 358178931.62457013, 358178931.62457013, 358767166.9186876], [0.016802055, 0.017660285, 0.017660285, 0.016802055, 0.016802055]}, {[646220455.0854722, 646220455.0854722], [0.01683985, 0.01694256]}, {[1407289616.8067927, 1407614578.9881935], [0.016892585, 0.017096840000000002]}, {[1109641333.4381282, 1109956422.4903247], [0.016968125, 0.017308995]}, {[1737912209.7280185, 1737912209.7280185, 1737388649.5185945, 1737388649.5185945, 1737912209.7280185], [0.01703635, 0.017548249999999998, 0.017548249999999998, 0.01703635, 0.01703635]}, {[649025150.3441954, 649025150.3441954, 648514946.2625628, 648514946.2625628, 649025150.3441954], [0.017075035, 0.017837065, 0.017837065, 0.017075035, 0.017075035]}, {[1368496775.7808926, 1368496775.7808926, 1367511554.106016, 1367511554.106016, 1368496775.7808926], [0.017146785, 0.017292625000000002, 0.017292625000000002, 0.017146785, 0.017146785]}, {[1739036854.6760328, 1739036854.6760328], [0.017148425, 0.017290769999999997]}, {[2549237037.2132626, 2549237037.2132626, 2549002570.624751, 2549002570.624751, 2549237037.2132626], [0.017206515, 0.01776483, 0.01776483, 0.017206515, 0.017206515]}, {[2603671203.2655973, 2603671203.2655973, 2603212487.669267, 2603212487.669267, 2603671203.2655973], [0.017252575, 0.017407765, 0.017407765, 0.017252575, 0.017252575]}, {[549553368.0452126, 549553368.0452126], [0.01731188, 0.017521340000000003]}, {[1450593739.7889042, 1450593739.7889042, 1450031942.0360951, 1450031942.0360951, 1450593739.7889042], [0.01737319, 0.01759628, 0.01759628, 0.01737319, 0.01737319]}, {[1925417085.794845, 1925417085.794845], [0.01737931, 0.01768643]}, {[1442895839.5533645, 1442895839.5533645, 1441826320.836787, 1441826320.836787, 1442895839.5533645], [0.017387375, 0.01745635, 0.01745635, 0.017387375, 0.017387375]}, {[2879644419.775343, 2879644419.775343], [0.01739394, 0.017468545]}, {[767371731.6235411, 767371731.6235411], [0.01747183, 0.01760342]}, {[285702284.61423993, 285848939.51949644], [0.017566925, 0.017644685]}, {[1663781411.623024, 1663781411.623024, 1662888554.480167, 1662888554.480167, 1663781411.623024], [0.01757235, 0.01778482, 0.01778482, 0.01757235, 0.01757235]}, {[1514007725.1357243, 1514007725.1357243, 1513539341.060783, 1513539341.060783, 1514007725.1357243], [0.01760568, 0.017834995, 0.017834995, 0.01760568, 0.01760568]}, {[1449379123.164526, 1449379123.164526, 1449227031.9097729, 1449227031.9097729, 1449379123.164526], [0.017669205, 0.017840565, 0.017840565, 0.017669205, 0.017669205]}, {[2800458079.9117093, 2800458079.9117093], [0.01768671, 0.01778528]}, {[734773527.9249377, 734773527.9249377], [0.0177003, 0.017884655]}, {[1662528595.771115, 1662528595.771115, 1662106654.842845, 1662106654.842845, 1662528595.771115], [0.01771909, 0.01805696, 0.01805696, 0.01771909, 0.01771909]}, {[1824904553.6381621, 1824904553.6381621, 1823914454.628261, 1823914454.628261, 1824904553.6381621], [0.01775116, 0.017827005, 0.017827005, 0.01775116, 0.01775116]}, {[2893767854.8132114, 2893767854.8132114], [0.01778056, 0.018020165]}, {[2773994345.1497536, 2773994345.1497536], [0.017806395, 0.017946885]}, {[1592242637.762581, 1592242637.762581], [0.01790229, 0.018069975000000002]}, {[2721608626.7745028, 2721608626.7745028, 2720795618.6444216, 2720795618.6444216, 2721608626.7745028], [0.01793453, 0.018111175, 0.018111175, 0.01793453, 0.01793453]}, {[2296778933.328233, 2296778933.328233], [0.017978005, 0.018083904999999997]}, {[1929892018.70746, 1930494645.6598828], [0.01797859, 0.01827535]}, {[1468527568.6407409, 1468752448.9319117], [0.018096275, 0.018305275]}, {[680656193.5764762, 680656193.5764762], [0.018109835, 0.01839423]}, {[1705890136.714889, 1705890136.714889, 1705866330.0252094, 1705866330.0252094, 1705890136.714889], [0.018136715, 0.01830276, 0.01830276, 0.018136715, 0.018136715]}, {[2203282501.0590725, 2203282501.0590725, 2202504290.942341, 2202504290.942341, 2203282501.0590725], [0.018153705, 0.01827362, 0.01827362, 0.018153705, 0.018153705]}, {[196366458.63001823, 197013797.4217322], [0.018203655, 0.018370314999999998]}, {[771488763.1909392, 772464303.5419035], [0.01824882, 0.01838292]}, {[2274485485.8791656, 2274697142.4636173], [0.018314195, 0.018392964999999997]}, {[2251875551.355018, 2251875551.355018, 2251530128.2116675, 2251530128.2116675, 2251875551.355018], [0.01833924, 0.018414335, 0.018414335, 0.01833924, 0.01833924]}, {[472589383.96592045, 472589383.96592045, 472241557.87896395, 472241557.87896395, 472589383.96592045], [0.018371595, 0.018534385, 0.018534385, 0.018371595, 0.018371595]}, {[2543674998.569998, 2543674998.569998], [0.018476845, 0.01862254]}, {[1631385191.5930405, 1631385191.5930405, 1630409581.836943, 1630409581.836943, 1631385191.5930405], [0.018555435, 0.018741055, 0.018741055, 0.018555435, 0.018555435]}, {[1684985896.9107437, 1684985896.9107437, 1684587490.5362415, 1684587490.5362415, 1684985896.9107437], [0.01858458, 0.018814215, 0.018814215, 0.01858458, 0.01858458]}, {[2865988826.0049314, 2865988826.0049314, 2865959435.8506327, 2865959435.8506327, 2865988826.0049314], [0.018666215, 0.01894171, 0.01894171, 0.018666215, 0.018666215]}, {[1580862112.1019201, 1580896379.0230677], [0.01877004, 0.01901347]}, {[740798571.8011333, 741021269.8056967], [0.01879697, 0.01896333]}, {[2151381942.365458, 2152309537.7059007], [0.018867985, 0.01898791]}, {[997414748.4713764, 997414748.4713764, 997259949.7097666, 997259949.7097666, 997414748.4713764], [0.01887159, 0.018931415, 0.018931415, 0.01887159, 0.01887159]}, {[1739062096.239286, 1739062096.239286], [0.019015335, 0.01915768]}, {[646574240.5246942, 646574240.5246942], [0.01906667, 0.01916938]}, {[1407325102.8832715, 1407650065.0646722], [0.01913829, 0.019342545]}, {[1367885637.5937536, 1367885637.5937536, 1366900415.9188766, 1366900415.9188766, 1367885637.5937536], [0.01919505, 0.019340890000000003, 0.019340890000000003, 0.01919505, 0.01919505]}, {[2879383848.0123553, 2879383848.0123553], [0.019227475, 0.01930208]}, {[826838300.9996495, 826838300.9996495, 826802029.6902552, 826802029.6902552, 826838300.9996495], [0.019238375, 0.0193881, 0.0193881, 0.019238375, 0.019238375]}, {[1038356381.8125423, 1038356381.8125423, 1037913903.936436, 1037913903.936436, 1038356381.8125423], [0.019315235, 0.01943497, 0.01943497, 0.019315235, 0.019315235]}, {[2681025969.7430334, 2681025969.7430334, 2679883112.6001763, 2679883112.6001763, 2681025969.7430334], [0.019326565, 0.01940584, 0.01940584, 0.019326565, 0.019326565]}, {[2754686769.2260327, 2754686769.2260327, 2754008803.1243377, 2754008803.1243377, 2754686769.2260327], [0.019340045, 0.01959207, 0.01959207, 0.019340045, 0.019340045]}, {[1442243301.1614661, 1442243301.1614661, 1441173782.4448886, 1441173782.4448886, 1442243301.1614661], [0.01934136, 0.019410334999999997, 0.019410334999999997, 0.01934136, 0.01934136]}, {[2383560511.0241203, 2383560511.0241203], [0.019356, 0.019674705]}, {[2880935289.150682, 2880935289.150682], [0.019479185, 0.019996925]}, {[2708542967.9208097, 2708542967.9208097, 2707742967.9208097, 2707742967.9208097, 2708542967.9208097], [0.01955157, 0.01979364, 0.01979364, 0.01955157, 0.01955157]}, {[549553368.0452126, 549553368.0452126], [0.01957761, 0.01978707]}, {[1824760819.596036, 1824760819.596036, 1823770720.586135, 1823770720.586135, 1824760819.596036], [0.019617395, 0.01969324, 0.01969324, 0.019617395, 0.019617395]}, {[1449313379.2357452, 1449313379.2357452, 1449161287.9809923, 1449161287.9809923, 1449313379.2357452], [0.019654225, 0.019825585, 0.019825585, 0.019654225, 0.019654225]}, {[1513974483.6750598, 1513974483.6750598, 1513506099.6001184, 1513506099.6001184, 1513974483.6750598], [0.019683485, 0.0199128, 0.0199128, 0.019683485, 0.019683485]}, {[1450668975.5348005, 1450668975.5348005, 1450107177.7819917, 1450107177.7819917, 1450668975.5348005], [0.019710445, 0.019933535, 0.019933535, 0.019710445, 0.019710445]}, {[2296419656.6224246, 2296419656.6224246], [0.019717075, 0.019822975]}, {[1489537063.0127218, 1489537063.0127218], [0.019719005, 0.019917425000000002]}, {[592275582.16434, 592275582.16434, 591126156.8769836, 591126156.8769836, 592275582.16434], [0.019734805, 0.020149725, 0.020149725, 0.019734805, 0.019734805]}, {[2845715761.121375, 2845715761.121375, 2845044620.181778, 2845044620.181778, 2845715761.121375], [0.0197504, 0.020042465000000002, 0.020042465000000002, 0.0197504, 0.0197504]}, {[1409155349.303642, 1409155349.303642, 1408497454.5667999, 1408497454.5667999, 1409155349.303642], [0.01978131, 0.020185075, 0.020185075, 0.01978131, 0.01978131]}, {[2395381985.8705244, 2395381985.8705244, 2395091288.196106, 2395091288.196106, 2395381985.8705244], [0.01978675, 0.020497599999999998, 0.020497599999999998, 0.01978675, 0.01978675]}, {[2642950869.969036, 2642950869.969036], [0.019819535, 0.020174809999999998]}, {[2721648319.4452286, 2721648319.4452286, 2720835311.3151474, 2720835311.3151474, 2721648319.4452286], [0.019871835, 0.02004848, 0.02004848, 0.019871835, 0.019871835]}, {[2402109882.815182, 2402175479.712059], [0.019892195, 0.020149390000000003]}, {[2800080381.365308, 2800080381.365308], [0.019928935, 0.020027504999999998]}, {[734464036.7508987, 734464036.7508987], [0.019959095, 0.02014345]}, {[1592373712.2870533, 1592373712.2870533], [0.019977005, 0.02014469]}, {[2603685887.7347784, 2603685887.7347784, 2603227172.1384487, 2603227172.1384487, 2603685887.7347784], [0.01998735, 0.02014254, 0.02014254, 0.01998735, 0.01998735]}, {[285702284.61423993, 285848939.51949644], [0.01999089, 0.02006865]}, {[1705556870.2031665, 1705556870.2031665, 1705533063.5134866, 1705533063.5134866, 1705556870.2031665], [0.01999527, 0.020161315, 0.020161315, 0.01999527, 0.01999527]}, {[196172012.7292211, 196819351.52093506], [0.02001107, 0.020177729999999998]}, {[771557701.0120342, 772533241.3629985], [0.020074505, 0.020208605]}, {[472872663.51137424, 472872663.51137424, 472524837.42441773, 472524837.42441773, 472872663.51137424], [0.02012252, 0.02028531, 0.02028531, 0.02012252, 0.02012252]}, {[2543843582.5957413, 2543843582.5957413], [0.02022938, 0.020375075000000003]}, {[348658294.97384024, 348658294.97384024, 347753317.5982747, 347753317.5982747, 348658294.97384024], [0.02024779, 0.02062173, 0.02062173, 0.02024779, 0.02024779]}, {[2893772879.06791, 2893772879.06791], [0.02029159, 0.020531195000000002]}, {[2274827967.994156, 2275039624.5786076], [0.02031984, 0.020398609999999998]}, {[1664115416.790714, 1664115416.790714, 1663222559.647857, 1663222559.647857, 1664115416.790714], [0.020400415, 0.020612885, 0.020612885, 0.020400415, 0.020400415]}, {[1925417085.794845, 1925417085.794845], [0.020406315, 0.020713435000000002]}, {[894525289.2485374, 894525289.2485374, 893461459.4613034, 893461459.4613034, 894525289.2485374], [0.02051478, 0.02107105, 0.02107105, 0.02051478, 0.02051478]}, {[1631342114.2469568, 1631342114.2469568, 1630366504.4908593, 1630366504.4908593, 1631342114.2469568], [0.0205785, 0.02076412, 0.02076412, 0.0205785, 0.0205785]}]
  in  "time range":cluster{"Numeric":dbl, "Numeric":dbl}(slide)={"Numeric"=0.0, "Numeric"=1181732.2396298076} scale=0.0..50.0 scale format="%#_6f"
  in  "refresh_file show":bool
  in  "color plate 2":T7={"PSK Color"=4591, "LFM Color"=16711680, "CW Color"=0}
  in  "Mode":T8(ring)=enum."5785 - 3.2GHz"
  out "Num of pulses":i32=1210602 format="%#.1p"
  in  "generate":bool=TRUE
  out "DDS free":bool[][](array[boolean])=[[FALSE, FALSE, FALSE], [FALSE, FALSE, FALSE], [FALSE, FALSE, FALSE], [FALSE, FALSE, FALSE], [FALSE, FALSE, FALSE], [FALSE, FALSE, FALSE], [TRUE, TRUE, TRUE], [TRUE, TRUE, TRUE], [TRUE, TRUE, TRUE], [TRUE, TRUE, TRUE], [TRUE, TRUE, TRUE], [TRUE, TRUE, TRUE], [TRUE, TRUE, TRUE], [TRUE, TRUE, TRUE], [TRUE, TRUE, TRUE], [TRUE, TRUE, TRUE]]
  in  "run it again when done":bool=TRUE
  in  "run":bool=TRUE
  # "Multi Emitter Generator"
  # "modulation \ntypes:"
  # "csv coloms:\nt_start(sec)\nf_Hz\nduration (sec)\namp(dB)\nmod type\nmod_depth (Hz)\ndiraction (deg)"
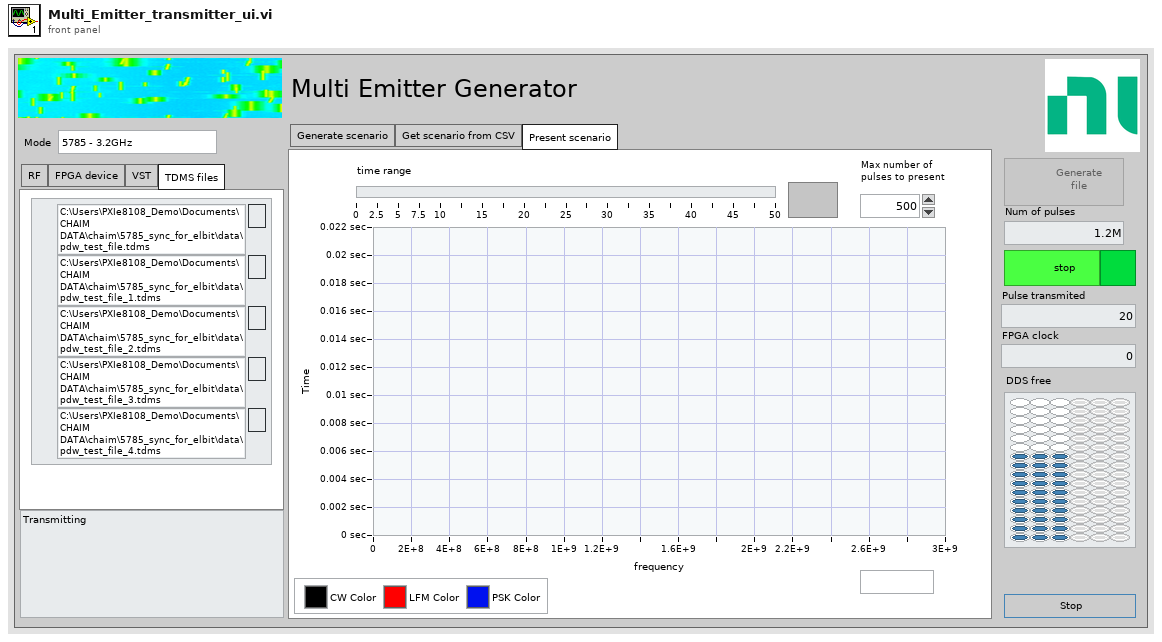
[diagram p1: front panel]
types:
  T1 = typedef "nirio_resource_hc.ctl" = tag
  T2 = enum32{"Generate scenario", "Get scenario from CSV", "Present scenario"}
  T3 = enum32{"Random emitters", "User specified emitters"}
  T4 = typedef "random_limits.ctl" = cluster{"# Number of emitters":u32, "# Number of frequency per emitter":cluster{"Numeric":u32, "Numeric":u32}, "Frequency range":cluster{"Numeric":dbl, "Numeric":dbl}, "Frequency dispersion for each emitter":cluster{"Numeric":dbl, "Numeric":dbl}, "PRI range (Hz)":cluster{"Numeric":dbl, "Numeric":dbl}, "Duty cycle - pulse in PRI":cluster{"Numeric":dbl, "Numeric":dbl}, "Amplitude (dB)":cluster{"Numeric":dbl, "Numeric":dbl}, "Modulation depth":cluster{"Numeric":dbl, "Numeric":dbl}, "CW":bool, "LFM":bool, "DOA (DEG)":cluster{"Numeric":dbl, "Numeric":dbl}, "start time (Sec)":dbl, "end time (Sec)":dbl, "BPSK":bool, "QPSK":bool}
  T5 = typedef "emitter params.ctl" = cluster{"f set":dbl[], "hop rate (Hz)":dbl, "d.c.":dbl, "amp (dB)":dbl, "mod type":T6, "mod depth":dbl, "DOA":dbl, "t start":dbl, "t end":dbl}
  T6 = typedef "mode_type.ctl" = enum8{"CW", "NC - CW", "NC - cw", "LFM", "BPSK", "QPSK"}
  T7 = cluster{"PSK Color":u32, "LFM Color":u32, "CW Color":u32}
  T8 = enum16{"USRP - 180MHz", "5785 - 2*180MHz", "5785 - 3.2GHz", "P2P - VST"}
  T9 = typedef "secnario config.ctl" = cluster{"devicess 2":T1[], "file paths":path[], "buffer size":u32, "Fs  FPGA":dbl, "SPC":dbl, "center frequency (Hz) ":dbl, "t clock ref":refnum<k20>[], "fpga rfe":refnum<k20>[], "tdms refs":refnum<k34>[], "niUsrpRio Session (out)":T10, "RF gain ":i32, "mode":u8, "vst_device":refnum<k15>[], "IQ_rare_p2p":dbl, "stream sesion P2P":refnum<k20>[]}
  T10 = typedef "niUsrpRio Config v1 Host.lvlib/niUsrpRio Session.ctl" = cluster{"FPGA Interface":refnum<k20>, "RIO Interface Number":u32, "Data Clock Rate":u32, "FPGA Data Clock Rate":u32, "Global Settings Register Bus":T11, "Radio 0 Settings Register Bus":T11, "Radio 1 Settings Register Bus":T11, "Radio Settings Bus Semaphore":T12, "DB Queues":T13[], "Characterization Data Valid?":bool, "EEPROM Header":T14, "Device Data Header":T15, "EEPROM Characterization Header":T16, "Characterization Data":T17[], "FPGA Current Version":u32, "FPGA Oldest Compatible Version":u32, "Fixed Logic Current Version":u32, "Fixed Logic Oldest Compatible Version":u32, "FPGA Radio Settings Bus Current Version":u32, "FPGA Radio Settings Bus Oldest Compatible Version":u32, "FPGA Board Config Current Version":u32, "FPGA Board Config Oldest Compatible Version":u32, "Daughterboard Clock Rate":u32, "daughterboard configuration session handles":u64[]}
  T11 = typedef "niInstr Register Bus v0 Host.lvlib/Register Bus Session.ctl" = refnum<queue>
  T12 = typedef "Semaphore RefNum" = refnum<k1>
  T13 = typedef "niUsrpRio Config v1 Host.lvlib/DB Queue Reference.ctl" = refnum<queue>
  T14 = typedef "niUsrpRio Config v1 Host.lvlib/EEPROM Header.ctl" = cluster{"Checksum":u32, "Product Code":u16, "Hardware Current Version":u16, "Hardware Oldest Compatible Version":u16, "EEPROM Map Current Version":u16, "EEPROM Map Oldest Compatible Version":u16, "User Password":string, "Pointer to Factory Header":u32, "Pointer to User Header":u32, "Recommended Interval":u16, "Number of Reserved Bytes":i32, "Number of Daughterboards":u8, "Daughterboard IDs":u16[], "Daughterboard Serial Numbers":string[]}
  T15 = typedef "niUsrpRio Config v1 Host.lvlib/EEPROM Device Data Header.ctl" = cluster{"Checksum":u32, "Number of Channels":u8, "Number of Gain Settings":u16[], "Pointer to Characterization Data":u32[], "Number of Reserved Bytes":i32, "Number of Frequencies":u16[]}
  T16 = typedef "niUsrpRio Config v1 Host.lvlib/EEPROM Characterization Header.ctl" = cluster{"Checksum":u32, "Date":timestamp, "Temperature":sgl, "Misc. Info":string, "Pointer to Device Data Header":u32, "Number of Reserved Bytes":i32}
  T17 = typedef "niUsrpRio Config v1 Host.lvlib/Characterization Data.ctl" = cluster{"Gains[dB]":dbl[], "Frequencies [Hz]":dbl[], "IQ Imbalance Table":T18[], "Measured Gains[dB]":dbl[][]}
  T18 = typedef "niUsrpRio Config v1 Host.lvlib/IQ Imbalance.ctl" = cluster{"Gain Imbalance [linear]":dbl, "Phase Imbalance [radians]":dbl, "Offset":cdb}
  T19 = cluster{"vst_device":refnum<k15>[], "RF gain ":dbl, "buffer size":u32, "center frequency (Hz) ":dbl, "P2P sample rate":dbl, "mode":enum16{"USRP - 180MHz", "5785 - 2*180MHz", "5785 - 3.2GHz", "P2P - VST"}, "devicess":T1[], "file paths":path[]}
  T20 = enum8{"Enabled", "Disabled", "Disabled and Grayed Out"}
  T21 = typedef "PDW_lv2.ctl" = cluster{"t start":dbl, "frequency (Hz)":dbl, "duration (sec)":dbl, "amp (lin)":dbl, "mod type":T6, "mod depth":dbl, "phase (rad)":dbl[]}
  T22 = typedef "pdw.ctl" = cluster{"PW":u32, "frequency shift":fxp<+/-,48,0>, "amp":fxp<+/-,18,1>, "mode type":T6, "mode depth":u32, "mode filter":u8, "phase shift":fxp<+/-,16,1>, "pulse shape filter":u8}
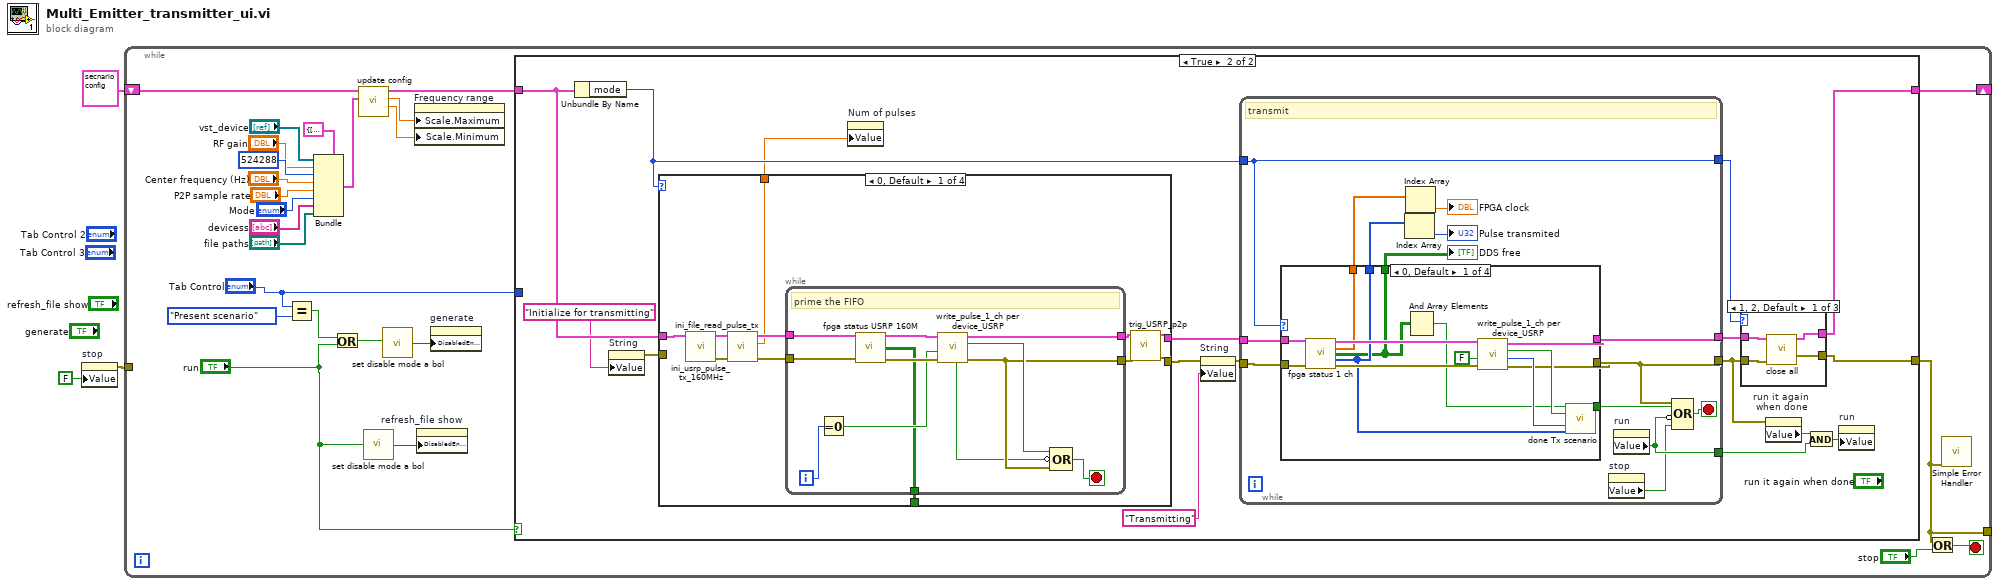
[diagram p0: block diagram]
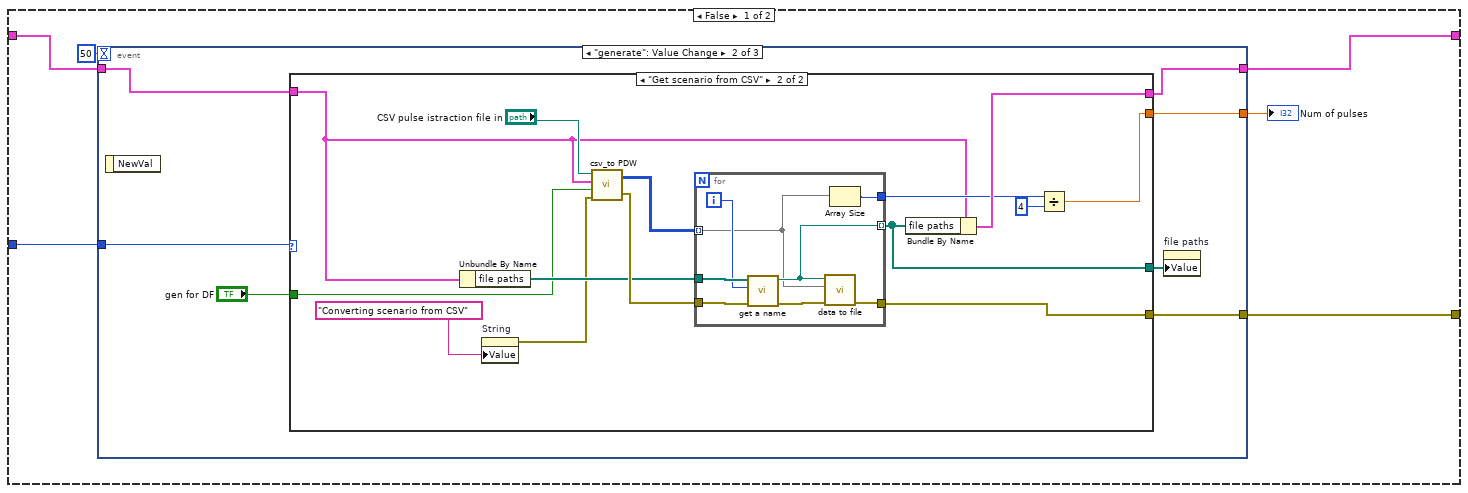
[diagram p2: hidden frame]
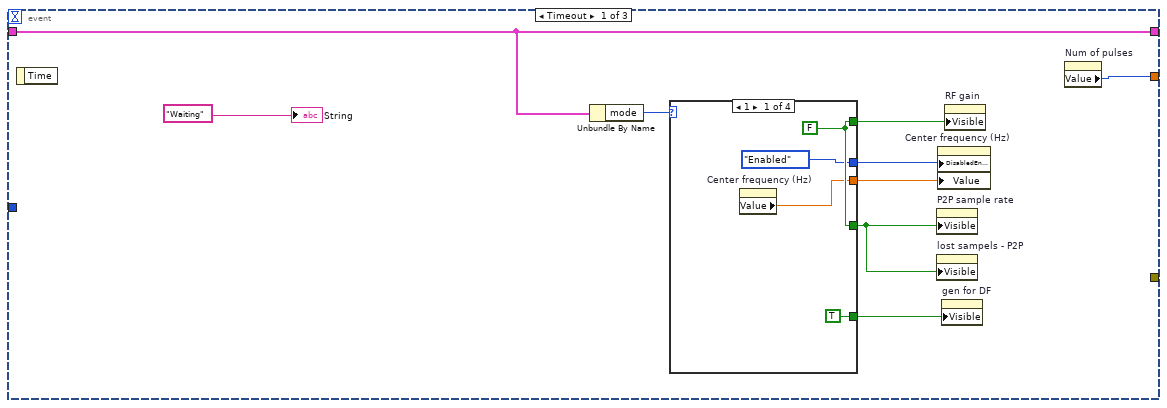
[diagram p3: hidden frame]
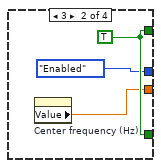
[diagram p4: hidden frame]
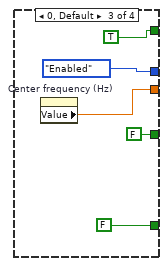
[diagram p5: hidden frame]
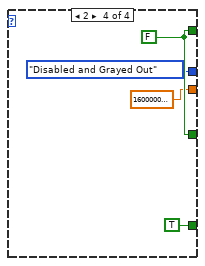
[diagram p6: hidden frame]
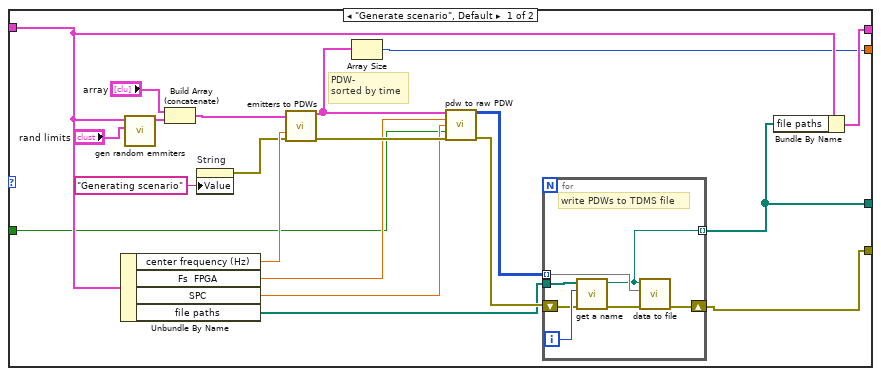
[diagram p7: hidden frame]
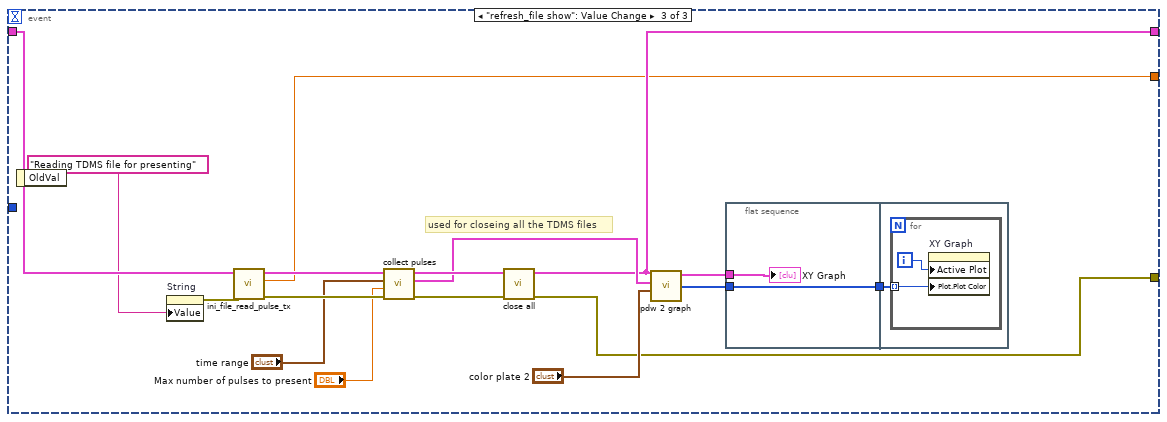
[diagram p8: hidden frame]
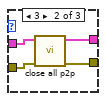
[diagram p9: hidden frame]
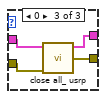
[diagram p10: hidden frame]
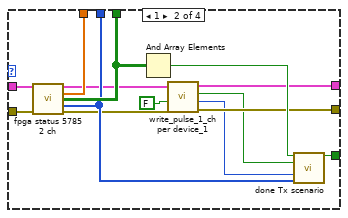
[diagram p11: hidden frame]
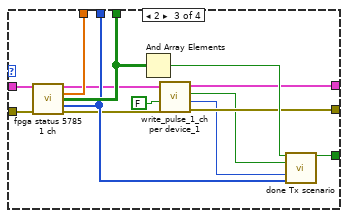
[diagram p12: hidden frame]
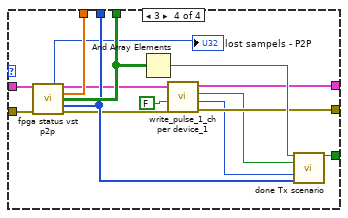
[diagram p13: hidden frame]
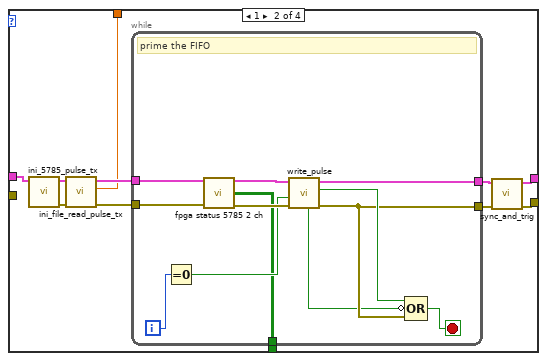
[diagram p14: hidden frame]
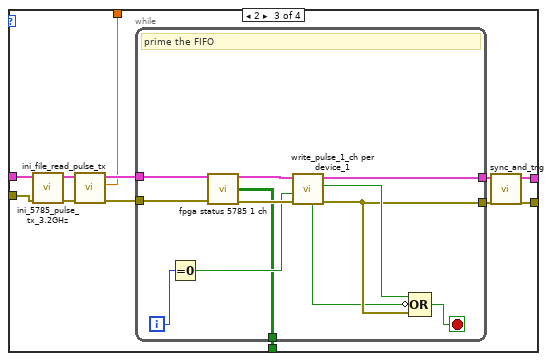
[diagram p15: hidden frame]
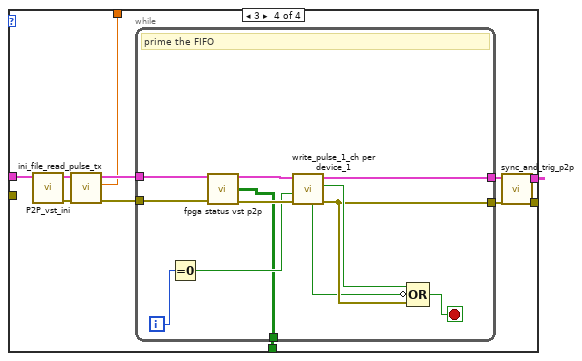
[diagram p16: hidden frame]
diagram:
  n1 = property on="stop" class="Bool (strict)"("Value"=FALSE ("stop")) -> (error out=w1:errorcluster)  [unwired: 2 in, 1 out]
  n2 = while {
    shift-right: [w16] -> _
    shift-left: T9 {"devicess 2"=["IF_transiver_1", "IF_transiver_2"], "file paths"=[path "C:/Users/PXIe8108_Demo/Documents/CHAIM DATA/chaim/5785_sync_for_elbit/data/pdw_test_file.tdms", path "C:/Users/PXIe8108_Demo/Documents/CHAIM DATA/chaim/5785_sync_for_elbit/data/pdw_test_file.tdms", path "C:/Users/PXIe8108_Demo/Documents/CHAIM DATA/chaim/5785_sync_for_elbit/data/pdw_test_file.tdms", path "C:/Users/PXIe8108_Demo/Documents/CHAIM DATA/chaim/5785_sync_for_elbit/data/pdw_test_file.tdms"], "buffer size"=524288, "Fs  FPGA"=200000000.0, "SPC"=1.0, "center frequency (Hz) "=1000000000.0, "t clock ref"=[], "fpga rfe"=[], "tdms refs"=[], "niUsrpRio Session (out)"={"FPGA Interface"=refnum, "RIO Interface Number"=0, "Data Clock Rate"=0, "FPGA Data Clock Rate"=0, "Global Settings Register Bus"=refnum, "Radio 0 Settings Register Bus"=refnum, "Radio 1 Settings Register Bus"=refnum, "Radio Settings Bus Semaphore"=refnum, "DB Queues"=[], "Characterization Data Valid?"=FALSE, "EEPROM Header"={"Checksum"=0, "Product Code"=0, "Hardware Current Version"=0, "Hardware Oldest Compatible Version"=0, "EEPROM Map Current Version"=0, "EEPROM Map Oldest Compatible Version"=0, "User Password"="", "Pointer to Factory Header"=0, "Pointer to User Header"=0, "Recommended Interval"=0, "Number of Reserved Bytes"=9, "Number of Daughterboards"=0, "Daughterboard IDs"=[], "Daughterboard Serial Numbers"=[]}, "Device Data Header"={"Checksum"=0, "Number of Channels"=0, "Number of Gain Settings"=[], "Pointer to Characterization Data"=[], "Number of Reserved Bytes"=27, "Number of Frequencies"=[]}, "EEPROM Characterization Header"={"Checksum"=0, "Date"=timestamp(0 s since 1904-01-01), "Temperature"=0.0, "Misc. Info"="", "Pointer to Device Data Header"=0, "Number of Reserved Bytes"=28}, "Characterization Data"=[], "FPGA Current Version"=0, "FPGA Oldest Compatible Version"=0, "Fixed Logic Current Version"=0, "Fixed Logic Oldest Compatible Version"=0, "FPGA Radio Settings Bus Current Version"=0, "FPGA Radio Settings Bus Oldest Compatible Version"=0, "FPGA Board Config Current Version"=0, "FPGA Board Config Oldest Compatible Version"=0, "Daughterboard Clock Rate"=0, "daughterboard configuration session handles"=[]}, "RF gain "=10, "mode"=2, "vst_device"=[], "IQ_rare_p2p"=200000000.0, "stream sesion P2P"=[]} ("secnario config") -> [w18]
    tunnel: [w10] -> _
    tunnel: w1 -> [_]
    stop <- w28 stop-if-true
    n3 = Equal?(x="Tab Control", y=T2."Present scenario") -> (x = y?=w7:bool)
    n4 = Bundle(cluster=T19 {"vst_device"=["VST_1", "VST_2"], "RF gain "=10.0, "buffer size"=524288, "center frequency (Hz) "=1000000000.0, "P2P sample rate"=200000000.0, "mode"=enum."5785 - 2*180MHz", "devicess"=["IF_transiver_0", "IF_transiver_1", "IF_transiver_2"], "file paths"=[path "C:/Users/PXIe8108_Demo/Documents/CHAIM DATA/chaim/5785_sync_for_elbit/data/pdw_test_file.tdms", path "C:/Users/PXIe8108_Demo/Documents/CHAIM DATA/chaim/5785_sync_for_elbit/data/pdw_test_file_1.tdms", path "C:/Users/PXIe8108_Demo/Documents/CHAIM DATA/chaim/5785_sync_for_elbit/data/pdw_test_file_2.tdms", path "C:/Users/PXIe8108_Demo/Documents/CHAIM DATA/chaim/5785_sync_for_elbit/data/pdw_test_file_3.tdms", path "C:/Users/PXIe8108_Demo/Documents/CHAIM DATA/chaim/5785_sync_for_elbit/data/pdw_test_file_4.tdms"]} ("user configurations"), "vst_device"="vst_device", "RF gain"="RF gain", "buffer size"=u32 524288, "center frequency (Hz)"="Center frequency (Hz)", "P2P sample rate"="P2P sample rate", "mode"="Mode", "devicess"="devicess", "file paths"="file paths") -> (w19:T19)
    n5 = Or(x=w7, y="run") -> (x .or. y?=w4:bool)
    n6 = call "update config.vi"("user configurations 2"=w19, "secnario config in"=w18) -> ("min frequency"=w11:dbl, "max frequency"=w12:dbl, "secnario config out"=w17:T9)  [unwired: 7 in]
    n7 = call "set disable mode a bol.vi"("run"="run") -> ("Disabled"=w15:T20)
    n8 = call "set disable mode a bol.vi"("run"=w4) -> ("Disabled"=w5:T20)
    n9 = property on="Frequency range" class="Slide (strict)"("Scale.Maximum"=w12, "Scale.Minimum"=w11) -> ()  [unwired: 2 in, 2 out]
    n10 = property on="refresh_file show" class="Bool (strict)"("DisabledEnum"=w15) -> ()  [unwired: 2 in, 2 out]
    n11 = property on="generate" class="Bool (strict)"("DisabledEnum"=w5) -> ()  [unwired: 2 in, 2 out]
    n12 = case shown="True" "run" {
      tunnel: w17 -> [w33 w154]
      tunnel: [w32 w150] -> w16
      tunnel: [w31 w149] -> w10
      tunnel: "Tab Control" -> [w29 _]
      frame False {
        n13 = event shown="[1] \"generate\": Value Change" {
          selector: _ -> [_ _ _]
          dyn-events: _ -> [_ _ _]
          timeout: 50 -> [_ _ _]
          tunnel: w33 -> [w38 w66 w123]
          tunnel: [w38 w64 w120] -> w32
          tunnel: [_ w63 w119] -> w31
          tunnel: [w43 w62 w118] -> w30
          tunnel: w29 -> [_ w60 _]
          event Timeout {
            n14 = event-data() -> ()  [unwired: 1 in, 1 out]
            n15 = Unbundle By Name(w38) -> ("mode"=w37:u8)
            n16 = case shown="1" w37 {
              tunnel: [w47 w50 TRUE ("Visible") w59] -> w39
              tunnel: [w47 w50 FALSE ("Visible") w59] -> w36
              tunnel: [T20."Enabled" ("Disabled") T20."Enabled" ("Disabled") T20."Enabled" ("Disabled") T20."Disabled and Grayed Out" ("Disabled")] -> w40
              tunnel: [w45 w48 w53 1600000000.0 ("center frequency (Hz)")] -> w41
              tunnel: [TRUE _ FALSE TRUE] -> w35
              frame 1 {
                w47 = FALSE ("Visible")
                n17 = property on="Center frequency (Hz)" class="DigNum (strict)"() -> ("Value"=w45:dbl)  [unwired: 2 in, 2 out]
              }
              frame 3 {
                w50 = TRUE ("Visible")
                n18 = property on="Center frequency (Hz)" class="DigNum (strict)"() -> ("Value"=w48:dbl)  [unwired: 2 in, 2 out]
              }
              frame 0, Default {
                n19 = property on="Center frequency (Hz)" class="DigNum (strict)"() -> ("Value"=w53:dbl)  [unwired: 2 in, 2 out]
              }
              frame 2 {
                w59 = FALSE ("Visible")
              }
            }
            n20 = property on="P2P sample rate" class="DigNum (strict)"("Visible"=w36) -> ()  [unwired: 2 in, 2 out]
            n21 = property on="lost sampels - P2P" class="DigNum (strict)"("Visible"=w36) -> ()  [unwired: 2 in, 2 out]
            n22 = property on="Center frequency (Hz)" class="DigNum (strict)"("DisabledEnum"=w40, "Value"=w41) -> ()  [unwired: 2 in, 2 out]
            n23 = property on="gen for DF" class="Bool (strict)"("Visible"=w35) -> ()  [unwired: 2 in, 2 out]
            n24 = property on="RF gain" class="DigNum (strict)"("Visible"=w39) -> ()  [unwired: 2 in, 2 out]
            n25 = property on="Num of pulses" class="DigNum (strict)"() -> ("Value"=w43:i32)  [unwired: 2 in, 2 out]
            "String" <- "Waiting" ("String")
          }
          event "generate": Value Change {
            n26 = event-data() -> ()  [unwired: 1 in, 1 out]
            n27 = case shown="\"Get scenario from CSV\"" w60 {
              tunnel: w66 -> [w76 w94]
              tunnel: "gen for DF" -> [w74 w104]
              tunnel: [w72 w102] -> w64
              tunnel: [w73 w101] -> w63
              tunnel: [w70 w98] -> w62
              tunnel: [w69 w97] -> w61
              frame "Generate scenario", Default {
                # "PDW- \nsorted by time"
                n28 = Unbundle By Name(w76) -> ("center frequency (Hz)"=w80:dbl, "Fs  FPGA"=w79:dbl, "SPC"=w78:dbl, "file paths"=w77:path[])
                n29 = call "gen random emmiters.vi"("rand limits"="rand limits", "secnario config"=w76) -> ("Array"=w86:T5[])  [unwired: 9 in]
                n30 = Build Array (concatenate)("array", w86) -> (w84:T5[])
                n31 = property on="String" class="Str"("Value"="Generating scenario" ("String")) -> (error out=w67:errorcluster)  [unwired: 2 in, 1 out]
                n32 = call "emitters to PDWs.vi"("emmiter"=w84, "center frequency (Hz)"=w80, "erorr in"=w67) -> ("sorted array"=w85:T21[], "erorr out"=w83:errorcluster)  [unwired: 10 in, 1 out]
                n33 = Array Size(array=w85) -> (size(s)=w70:i32)
                n34 = call "pdw to raw PDW.vi"("PDWs"=w85, "Fs fpGa"=w79, "SPC"=w78, "gen for DF"=w74, "erorr in"=w83) -> ("Array"=w81:u64[][], "erorr out"=w82:errorcluster)  [unwired: 8 in, 1 out]
                n35 = for {
                  tunnel: w77 -> [w91]
                  tunnel: w81 -> [w93] mode=indexing
                  tunnel: [w88] -> w69 mode=indexing
                  shift-right: [w92] -> w73
                  shift-left: w82 -> [w89]
                  i -> [w90]
                  # "write PDWs to TDMS file"
                  n36 = call "get a name.vi"("error constant"=w89, "Numeric"=w90, "tdms pulse istraction file in"=w91) -> ("error constant 2"=w87:errorcluster, "Path"=w88:path)  [unwired: 7 in]
                  n37 = call "data to file.vi"("error in (no error)"=w87, "Array"=w93, "Path"=w88) -> ("error out"=w92:errorcluster)  [unwired: 8 in]
                }
                n38 = Bundle By Name(cluster=w76, "file paths"=w69) -> (w72:T9)
              }
              frame "Get scenario from CSV" {
                n39 = Unbundle By Name(w94) -> ("file paths"=w105:path[])
                n40 = property on="String" class="Str"("Value"="Converting scenario from CSV" ("String")) -> (error out=w95:errorcluster)  [unwired: 2 in, 1 out]
                n41 = call "csv_to PDW.vi"("error in (no error)"=w95, "gen for DF"=w104, "secnario config"=w94, "CSV file path (dialog if empty)"="CSV pulse istraction file in") -> ("error out"=w106:errorcluster, "u64_PDW"=w107:u64[][])
                n42 = for {
                  tunnel: w105 -> [w115]
                  tunnel: w107 -> [w109] mode=indexing
                  tunnel: w106 -> [w113]
                  tunnel: [w110] -> w97 mode=indexing
                  tunnel: [w111] -> w101
                  tunnel: [w108] -> w100
                  i -> [w114]
                  n43 = call "get a name.vi"("error constant"=w113, "Numeric"=w114, "tdms pulse istraction file in"=w115) -> ("error constant 2"=w112:errorcluster, "Path"=w110:path)  [unwired: 7 in]
                  n44 = call "data to file.vi"("error in (no error)"=w112, "Array"=w109, "Path"=w110) -> ("error out"=w111:errorcluster)  [unwired: 8 in]
                  n45 = Array Size(array=w109) -> (size(s)=w108:i32)
                }
                n46 = Bundle By Name(cluster=w94, "file paths"=w97) -> (w102:T9)
                n47 = Divide(x=w100, y=4) -> (x/y=w98:dbl)
              }
            }
            n48 = property on="file paths" class="Arr (strict)"("Value"=w61) -> ()  [unwired: 2 in, 2 out]
          }
          event "refresh_file show": Value Change {
            # "used for closeing all the TDMS files"
            n49 = event-data() -> ()  [unwired: 1 in, 1 out]
            n50 = property on="String" class="Str"("Value"="Reading TDMS file for presenting" ("String")) -> (error out=w116:errorcluster)  [unwired: 2 in, 1 out]
            n51 = call "ini_file_read_pulse_tx.vi"("error in (no error)"=w116, "secnario config"=w123) -> ("error out"=w130:errorcluster, "num pulses in file"=w118:dbl, "output cluster"=w128:T9)  [unwired: 7 in]
            n52 = call "collect pulses.vi"("error in (no error)"=w130, "max number of pulses to show"="Max number of pulses to present", "time range"="time range", "secnario config"=w128) -> ("error out"=w129:errorcluster, "PDW"=w126:cluster{"PDW":T22[], "Ton":dbl[]}, "secnario config"=w127:T9)  [unwired: 5 in]
            n53 = call "close all.vi"("error in (no error)"=w129, "secnario config in"=w127) -> ("error out"=w119:errorcluster, "secnario config"=w120:T9)  [unwired: 8 in]
            n54 = call "pdw 2 graph.vi"("color plate"="color plate 2", "PDW"=w126, "secnario config"=w120) -> ("color"=w131:u32[], "graph"=w125:cluster{dbl[], dbl[]}[])  [unwired: 7 in]
            n55 = flat-sequence {
              tunnel: w131 -> [w134]
              tunnel: [w134] -> w132
              tunnel: w125 -> [w133]
              tunnel: w132 -> [w135]
              frame #0 {
                "XY Graph" <- w133
              }
              frame #1 {
                n56 = for {
                  tunnel: w135 -> [w136] mode=indexing
                  i -> [w137]
                  n57 = property on="XY Graph" class="XYGraph (strict)"("Active Plot"=w137, "Plot.Plot Color"=w136) -> ()  [unwired: 2 in, 2 out]
                }
              }
            }
          }
        }
        "Num of pulses" <- w30
      }
      frame True {
        n58 = Unbundle By Name(w154) -> ("mode"=w152:u8)
        n59 = property on="String" class="Str"("Value"="Initialize for transmitting" ("String")) -> (error out=w141:errorcluster)  [unwired: 2 in, 1 out]
        n60 = case shown="0, Default" w152 {
          tunnel: w154 -> [w242 w270 w289 w312]
          tunnel: [w241 w264 w288 w311] -> w153
          tunnel: [w240 w263 w287 w310] -> w140
          tunnel: [w239 w262 w286 w309] -> _
          tunnel: [w238 w261 w285 w308] -> w143
          tunnel: w141 -> [_ _ w284 _]
          frame 0, Default {
            n61 = call "ini_usrp_pulse_tx_160MHz.vi"("secnario config"=w242) -> ("error out"=w248:errorcluster, "secnario config"=w247:T9)  [unwired: 9 in]
            n62 = call "ini_file_read_pulse_tx.vi"("error in (no error)"=w248, "secnario config"=w247) -> ("error out"=w245:errorcluster, "num pulses in file"=w238:dbl, "output cluster"=w246:T9)  [unwired: 7 in]
            n63 = while {
              tunnel: w246 -> [w260]
              tunnel: w245 -> [w259]
              tunnel: [w255] -> w244
              tunnel: [w252] -> w243
              tunnel: [w249] -> w239
              i -> [w258]
              stop <- w251 stop-if-true
              # "prime the FIFO"
              n64 = Equal To 0?(x=w258) -> (x = 0?=w254:bool)
              n65 = call "fpga status USRP 160M.vi"("secnario config"=w260, "error in (no error)"=w259) -> ("secnario config"=w257:T9, "dds free"=w249:bool[][], "error out"=w256:errorcluster)  [unwired: 9 in, 2 out]
              n66 = call "write_pulse_1_ch per device_USRP.vi"("error in"=w256, "first call"=w254, "secnario config"=w257) -> ("error out"=w252:errorcluster, "done write files"=w253:bool, "output cluster"=w255:T9, "room on the FIFO"=w250:bool)  [unwired: 4 in, 1 out]
              n67 = Compound Arithmetic op=OR(w253, invert w250, w252) -> (w251:bool)
            }
            n68 = call "trig_USRP_p2p.vi"("error in (no error)"=w243, "secnario config"=w244) -> ("error out"=w240:errorcluster, "secnario config 2"=w241:T9)  [unwired: 8 in]
          }
          frame 1 {
            n69 = call "ini_5785_pulse_tx.vi"("secnario config 2"=w270) -> ("error out"=w271:errorcluster, "secnario config"=w269:T9)  [unwired: 9 in]
            n70 = call "ini_file_read_pulse_tx.vi"("error in (no error)"=w271, "secnario config"=w269) -> ("error out"=w267:errorcluster, "num pulses in file"=w261:dbl, "output cluster"=w268:T9)  [unwired: 7 in]
            n71 = while {
              tunnel: w268 -> [w283]
              tunnel: w267 -> [w282]
              tunnel: [w278] -> w266
              tunnel: [w275] -> w265
              tunnel: [w272] -> w262
              i -> [w281]
              stop <- w274 stop-if-true
              # "prime the FIFO"
              n72 = Equal To 0?(x=w281) -> (x = 0?=w277:bool)
              n73 = call "fpga status 5785 2 ch.vi"("secnario config"=w283, "error in (no error)"=w282) -> ("secnario config"=w280:T9, "dds free"=w272:bool[][], "error out"=w279:errorcluster)  [unwired: 9 in, 2 out]
              n74 = call "write_pulse.vi"("error in"=w279, "first call"=w277, "secnario config"=w280) -> ("error out"=w275:errorcluster, "done write files"=w276:bool, "output cluster"=w278:T9, "room on the FIFO"=w273:bool)  [unwired: 4 in, 1 out]
              n75 = Compound Arithmetic op=OR(w276, invert w273, w275) -> (w274:bool)
            }
            n76 = call "sync_and_trig.vi"("error in (no error)"=w265, "secnario config"=w266) -> ("error out"=w263:errorcluster, "secnario config 2"=w264:T9)  [unwired: 8 in]
          }
          frame 2 {
            n77 = call "ini_5785_pulse_tx_3.2GHz.vi"("error in (no error)"=w284, "secnario config"=w289) -> ("error out"=w295:errorcluster, "secnario config"=w294:T9)  [unwired: 8 in]
            n78 = call "ini_file_read_pulse_tx.vi"("error in (no error)"=w295, "secnario config"=w294) -> ("error out"=w292:errorcluster, "num pulses in file"=w285:dbl, "output cluster"=w293:T9)  [unwired: 7 in]
            n79 = while {
              tunnel: w293 -> [w307]
              tunnel: w292 -> [w306]
              tunnel: [w302] -> w291
              tunnel: [w299] -> w290
              tunnel: [w296] -> w286
              i -> [w305]
              stop <- w298 stop-if-true
              # "prime the FIFO"
              n80 = Equal To 0?(x=w305) -> (x = 0?=w301:bool)
              n81 = call "fpga status 5785 1 ch.vi"("secnario config"=w307, "error in (no error)"=w306) -> ("secnario config"=w304:T9, "dds free"=w296:bool[][], "error out"=w303:errorcluster)  [unwired: 9 in, 2 out]
              n82 = call "write_pulse_1_ch per device_1.vi"("error in"=w303, "first call"=w301, "secnario config"=w304) -> ("error out"=w299:errorcluster, "done write files"=w300:bool, "output cluster"=w302:T9, "room on the FIFO"=w297:bool)  [unwired: 4 in, 1 out]
              n83 = Compound Arithmetic op=OR(w300, invert w297, w299) -> (w298:bool)
            }
            n84 = call "sync_and_trig.vi"("error in (no error)"=w290, "secnario config"=w291) -> ("error out"=w287:errorcluster, "secnario config 2"=w288:T9)  [unwired: 8 in]
          }
          frame 3 {
            n85 = call "P2P_vst_ini.vi"("secnario config"=w312) -> ("error out"=w318:errorcluster, "secnario config"=w317:T9)  [unwired: 9 in]
            n86 = call "ini_file_read_pulse_tx.vi"("error in (no error)"=w318, "secnario config"=w317) -> ("error out"=w315:errorcluster, "num pulses in file"=w308:dbl, "output cluster"=w316:T9)  [unwired: 7 in]
            n87 = while {
              tunnel: w316 -> [w330]
              tunnel: w315 -> [w329]
              tunnel: [w325] -> w314
              tunnel: [w322] -> w313
              tunnel: [w319] -> w309
              i -> [w328]
              stop <- w321 stop-if-true
              # "prime the FIFO"
              n88 = Equal To 0?(x=w328) -> (x = 0?=w324:bool)
              n89 = call "fpga status vst p2p.vi"("secnario config"=w330, "error in (no error)"=w329) -> ("secnario config"=w327:T9, "dds free"=w319:bool[][], "error out"=w326:errorcluster)  [unwired: 8 in, 3 out]
              n90 = call "write_pulse_1_ch per device_1.vi"("error in"=w326, "first call"=w324, "secnario config"=w327) -> ("error out"=w322:errorcluster, "done write files"=w323:bool, "output cluster"=w325:T9, "room on the FIFO"=w320:bool)  [unwired: 4 in, 1 out]
              n91 = Compound Arithmetic op=OR(w323, invert w320, w322) -> (w321:bool)
            }
            n92 = call "sync_and_trig_p2p.vi"("error out 2"=w313, "secnario config"=w314) -> ("error out"=w310:errorcluster, "secnario config 2"=w311:T9)  [unwired: 8 in]
          }
        }
        n93 = property on="Num of pulses" class="DigNum (strict)"("Value"=w143) -> ()  [unwired: 2 in, 2 out]
        n94 = property on="String" class="Str"(error in=w140, "Value"="Transmitting" ("String")) -> (error out=w139:errorcluster)  [unwired: 1 in, 1 out]
        n95 = while {
          tunnel: [w177] -> w151
          tunnel: w139 -> [w180]
          tunnel: [w175] -> w147
          tunnel: w153 -> [w176]
          tunnel: w152 -> [w174]
          tunnel: [w174] -> w148
          tunnel: [w173] -> w145
          stop <- w178 stop-if-true
          # "transmit"
          n96 = case shown="0, Default" w174 {
            tunnel: w180 -> [w187 w208 w222 w237]
            tunnel: [w181 w206 w220 w235] -> w179
            tunnel: [w184 w205 w219 w234] -> w168
            tunnel: [w185 w204 w218 w233] -> w172
            tunnel: [w186 w202 w216 w231] -> w171
            tunnel: [w182 w200 w214 w229] -> w177
            tunnel: [w183 w199 w213 w228] -> w175
            tunnel: w176 -> [w188 w195 w209 w224]
            frame 0, Default {
              n97 = call "fpga status 1 ch.vi"("secnario config"=w188, "error in (no error)"=w187) -> ("secnario config"=w192:T9, "fpga clock"=w186:dbl[], "dds free"=w184:bool[][], "pulse transmitted"=w185:u32[], "error out"=w191:errorcluster)  [unwired: 9 in]
              n98 = And Array Elements(Boolean array=w184) -> (logical AND=w190:bool)
              n99 = call "write_pulse_1_ch per device_USRP.vi"("error in"=w191, "first call"=FALSE, "secnario config"=w192) -> ("error out"=w183:errorcluster, "num of pulse sent to fpga"=w193:i32, "done write files"=w194:bool, "output cluster"=w182:T9)  [unwired: 4 in, 1 out]
              n100 = call "done Tx scenario.vi"("all dds free"=w190, "done write files"=w194, "num of pulse sent to fpga"=w193, "pulse transmitted"=w185) -> ("Checkbox out"=w181:bool)  [unwired: 11 in]
            }
            frame 1 {
              n101 = call "fpga status 5785 2 ch.vi"("secnario config"=w195, "error in (no error)"=w208) -> ("secnario config"=w201:T9, "fpga clock"=w202:dbl[], "dds free"=w205:bool[][], "pulse transmitted"=w204:u32[], "error out"=w203:errorcluster)  [unwired: 9 in]
              n102 = And Array Elements(Boolean array=w205) -> (logical AND=w207:bool)
              n103 = call "write_pulse_1_ch per device_1.vi"("error in"=w203, "first call"=FALSE, "secnario config"=w201) -> ("error out"=w199:errorcluster, "num of pulse sent to fpga"=w198:i32, "done write files"=w196:bool, "output cluster"=w200:T9)  [unwired: 4 in, 1 out]
              n104 = call "done Tx scenario.vi"("all dds free"=w207, "done write files"=w196, "num of pulse sent to fpga"=w198, "pulse transmitted"=w204) -> ("Checkbox out"=w206:bool)  [unwired: 11 in]
            }
            frame 2 {
              n105 = call "fpga status 5785 1 ch.vi"("secnario config"=w209, "error in (no error)"=w222) -> ("secnario config"=w215:T9, "fpga clock"=w216:dbl[], "dds free"=w219:bool[][], "pulse transmitted"=w218:u32[], "error out"=w217:errorcluster)  [unwired: 9 in]
              n106 = And Array Elements(Boolean array=w219) -> (logical AND=w221:bool)
              n107 = call "write_pulse_1_ch per device_1.vi"("error in"=w217, "first call"=FALSE, "secnario config"=w215) -> ("error out"=w213:errorcluster, "num of pulse sent to fpga"=w212:i32, "done write files"=w210:bool, "output cluster"=w214:T9)  [unwired: 4 in, 1 out]
              n108 = call "done Tx scenario.vi"("all dds free"=w221, "done write files"=w210, "num of pulse sent to fpga"=w212, "pulse transmitted"=w218) -> ("Checkbox out"=w220:bool)  [unwired: 11 in]
            }
            frame 3 {
              n109 = call "fpga status vst p2p.vi"("secnario config"=w224, "error in (no error)"=w237) -> ("lost sampels"=→"lost sampels - P2P":u32, "secnario config"=w230:T9, "fpga clock"=w231:dbl[], "dds free"=w234:bool[][], "pulse transmitted"=w233:u32[], "error out"=w232:errorcluster)  [unwired: 8 in]
              n110 = And Array Elements(Boolean array=w234) -> (logical AND=w236:bool)
              n111 = call "write_pulse_1_ch per device_1.vi"("error in"=w232, "first call"=FALSE, "secnario config"=w230) -> ("error out"=w228:errorcluster, "num of pulse sent to fpga"=w227:i32, "done write files"=w225:bool, "output cluster"=w229:T9)  [unwired: 4 in, 1 out]
              n112 = call "done Tx scenario.vi"("all dds free"=w236, "done write files"=w225, "num of pulse sent to fpga"=w227, "pulse transmitted"=w233) -> ("Checkbox out"=w235:bool)  [unwired: 11 in]
            }
          }
          "DDS free" <- w168
          n113 = Index Array(array=w172) -> (element=→"Pulse transmited":u32)  [unwired: 1 in]
          n114 = Index Array(array=w171) -> (element=→"FPGA clock":dbl)  [unwired: 1 in]
          n115 = property on="stop" class="Bool (strict)"() -> ("Value"=w167:bool)  [unwired: 2 in, 2 out]
          n116 = property on="run" class="Bool (strict)"() -> ("Value"=w173:bool)  [unwired: 2 in, 2 out]
          n117 = Compound Arithmetic op=OR(w175, w179, invert w173, w167) -> (w178:bool)
        }
        n118 = case shown="1, 2, Default" w148 {
          tunnel: w147 -> [w158 w162 w166]
          tunnel: [w157 w160 w165] -> w149
          tunnel: w151 -> [w156 w161 w164]
          tunnel: [w155 w159 w163] -> w150
          frame 1, 2, Default {
            n119 = call "close all.vi"("error in (no error)"=w158, "secnario config in"=w156) -> ("error out"=w157:errorcluster, "secnario config"=w155:T9)  [unwired: 8 in]
          }
          frame 3 {
            n120 = call "close all p2p.vi"("error in (no error)"=w162, "secnario config in"=w161) -> ("error out"=w160:errorcluster, "secnario config"=w159:T9)  [unwired: 8 in]
          }
          frame 0 {
            n121 = call "close all_ usrp.vi"("error in (no error)"=w166, "secnario config in"=w164) -> ("error out"=w165:errorcluster, "secnario config in 2"=w163:T9)  [unwired: 8 in]
          }
        }
        n122 = property on="run it again\n when done" class="Bool (strict)"(error in=w147) -> ("Value"=w146:bool)  [unwired: 1 in, 2 out]
        n123 = And(x=w146, y=w145) -> (x .and. y?=w144:bool)
        n124 = property on="run" class="Bool (strict)"("Value"=w144) -> ()  [unwired: 2 in, 2 out]
      }
    }
    n125 = Or(x=w10, y="stop") -> (x .or. y?=w28:bool)
    n126 = call <vilib>:"Simple Error Handler.vi"("error in (no error)"=w10) -> ()  [unwired: 4 in, 5 out]
  }
